vi "eyecat MAX v02_JS_140210.vi"() -> ()   [LabVIEW 2014]
doc: "This VI is an upgrade from the WIN 1_v4 that implements the ageing subrutine"
uses:
  Buttons/String output.ctl
  <vilib>/Utility/miscctls.llb/LVRowAndColumnTypeDef.ctl
  Buttons/Numeric control.ctl
  Buttons/String input.ctl
  Buttons/Numeric indicator.ctl
  Controls Win/Control 3.ctl
  <vilib>/Platform/TimedLoop/XDataNode/nitl_modes.ctl
  <vilib>/Platform/TimedLoop/XDataNode/timing_clust.ctl
  <vilib>/Platform/TimedLoop/XDataNode/wakeup.ctl
  <vilib>/Utility/file.llb/Read From Spreadsheet File (DBL).vi
  <vilib>/Utility/file.llb/Write To Spreadsheet File (string).vi
  <vilib>/Utility/file.llb/Read From Spreadsheet File (string).vi
  <vilib>/regexp/Match Regular Expression.xnode
  <vilib>/Platform/TimedLoop/XDataNode/XDataNode.xnode
  <vilib>/Platform/TimedLoop/XDataNode/XDNodeRunTimeDep.lvlib
panel:
  out "HC Cyc 2 Array":dbl[](array[numeric])
  out "SO Valve 2 array":dbl[](array[numeric])
  out "SO Valve 1 array":dbl[](array[numeric])
  out "Air Bal array":dbl[](array[numeric])
  out "HC Bal array":dbl[](array[numeric])
  out "Air Cyc array":dbl[](array[numeric])
  out "HC Cyc array":dbl[](array[numeric])
  out "File name":string
  out "Log?":bool
  out "Advanced Logging":bool
  out "output cluster":T2
  out "Connected":bool
  out "MKS 1":i16
  out "MKS 2":i16
  out "Furnace temp 2":dbl
  out "Full system?":bool
  out "Log interval (seconds)":T1
  in  "Flow rate Age":dbl
  in  "Inlet temp Age":dbl
  out "Stopped?":bool
  in  "Stop Cmd":T1
  out "Connected?":bool
  out "Error":dbl
  out "Iteration Duration":i64
  out "Finished Late? [i-1]":bool
  in  "stop TCP":bool
  in  "SO2 ppm":dbl
  out "Furnace temp 1":dbl
  out "stop 2":bool
  in  "Enum 1":i16=1
  in  "Acknowledge":bool
  out "Test number":u16
  out "Flag1":bool=TRUE
  out "EditPos Subc":T3
  out "Flag 2":bool=TRUE
  in  "Tab Control":T4(tab)
  out "Doors Unlocked":bool
  in  "Temperature Limit (°C)":T1=800.0 min=0.0 max=1200.0 step=1.0
  in  "Log Test Button":bool
  in  "File Name":T5="Test"
  in  "File Path":path=path "C:/DATA LOG"
  out "Fail":bool
  out "Pass":bool
  in  "Select Test Type":T6(radio)
  out "Standby":bool
  out "Doors Open":bool
  out "Extractor Fan On":bool
  out "Test In Progress":bool
  out "Cool Down":bool
  out "System Alarm":bool
  in  "Execute Leak Test Button":bool
  in  "Stop Test Button":bool
  in  "Start Test Button":bool
  in  "Advanced settings":bool
  in  "Inlet Temperature (°C)":T1=400.0 min=350.0 max=1000.0 step=1.0
  in  "Inlet LAMBDA Rich":T1=0.9 min=0.85 max=0.96 step=0.001
  in  "Inlet LAMBDA Lean":T1=1.2 min=1.02 max=3.0 step=0.001
  in  "Test Stop temperature (°C)":T1=300.0 min=100.0 max=1000.0 step=1.0
  in  "Test Start Temperature (°C)":T1=125.0 min=0.0 max=500.0 step=1.0
  in  "Furnace Ramp Rate (°C/min)":T1=15.0 min=1.0 max=50.0 step=0.1
  in  "NO:CO Ratio":T1=1.1 min=1.0 max=5.0 step=0.1
  in  "Inlet O2 (%)":T1=0.5 min=0.0 max=14.0 step=0.01
  in  "Inlet LAMBDA":T1=1.0 min=0.6 max=3.0 step=0.001
  out "Space Velocity (h-1)":T7
  out "Vol Flow @ STP (l/min)":T7
  in  "Test Flow Rate(g/s)":T1 min=0.0 max=100.0 step=0.01
  out "Sample Volume (litres)":T7
  in  "Number of Samples":T1=1.0 min=1.0 max=6.0 step=1.0
  in  "Sample Diameter (mm)":T1
  out "CO Theory (%)":T7 format="%#_3g"
  out "CO Theory (%)":T7 format="%#_3g"
  out "HC Theory (%)":T7
  in  "Sample Length (mm)":T1 min=0.0 step=0.5
  in  "NO ppm SW":dbl=500.0 caption="NO (ppm)" min=0.0 max=500.0 step=1.0
  in  "NO ppm Loff":T1 caption="NO ppm"
  in  "Delete sCycle":bool
  in  "Load sCycle":bool
  in  "Save sCycle":bool
  in  "Clear subcycle":bool
  in  "Clear Cycle Pattern":bool
  in  "Save Cycle":bool
  in  "Load Cycle":bool
  in  "Delete Cycle":bool
  out "Test Compiled":bool
  in  "Compile Test Button":bool
  in  "Sub-Cycle List":i32(listbox)=1
  in  "Cycle List":i32(listbox)=2
  out "Total Test Duration (hrs)":T8
  in  "Ageing Gas":enum32{"Radio Selection 1", "Radio Selection 2"}(radio)
  in  "Sub-Cycle Pattern":string[][](table) caption="Subcycle pattern"
  in  "Total Number of Cycles":T1=1.0 min=1.0 max=10000.0 step=1.0
  in  "Cycle Pattern":string[][](table)
  in  "Sub-Cycle Name":T5
  in  "Cycle Name":T5
  out "Heat Exchanger Temperatures (°C)":dynamicdata(graph)
  out "Flow Rate (g/s)":dynamicdata(graph)
  out "Sample Temperatures (°C)":dynamicdata(graph)
  out "System Temperatures (°C)":dynamicdata(graph)
  out "HC Concentration (ppm)":dynamicdata(graph)
  out "Lambda":dynamicdata(graph)
  out "M584L Upstream & Downstream":dynamicdata(graph)
  out "NO Concentration (ppm)":dynamicdata(graph)
  in  "Purge System":bool
  in  "Alarm ack":bool
  in  "Clear log":bool
  out "Table":string[][](table)
  out "Soft Alarm":bool
  out "Hard Alarm":bool
  # "Test Type"
  # "Test Commands"
  # "System Indicators"
  # "Leak Test"
  # "Catalyst Specification"
  # "Lightoff Settings"
  # "Furnace Lightoff Settings"
  # "Sweep Settings"
  # "CO/HC Lightoff Settings"
  # "0.96 < lambda < 0.85"
  # "1.02< lambda < 1.6"
  # "350 < Tinlet < 1000"
  # "NO Lightoff Settings"
  # "Flow Specification"
  # "Cycle Compiled"
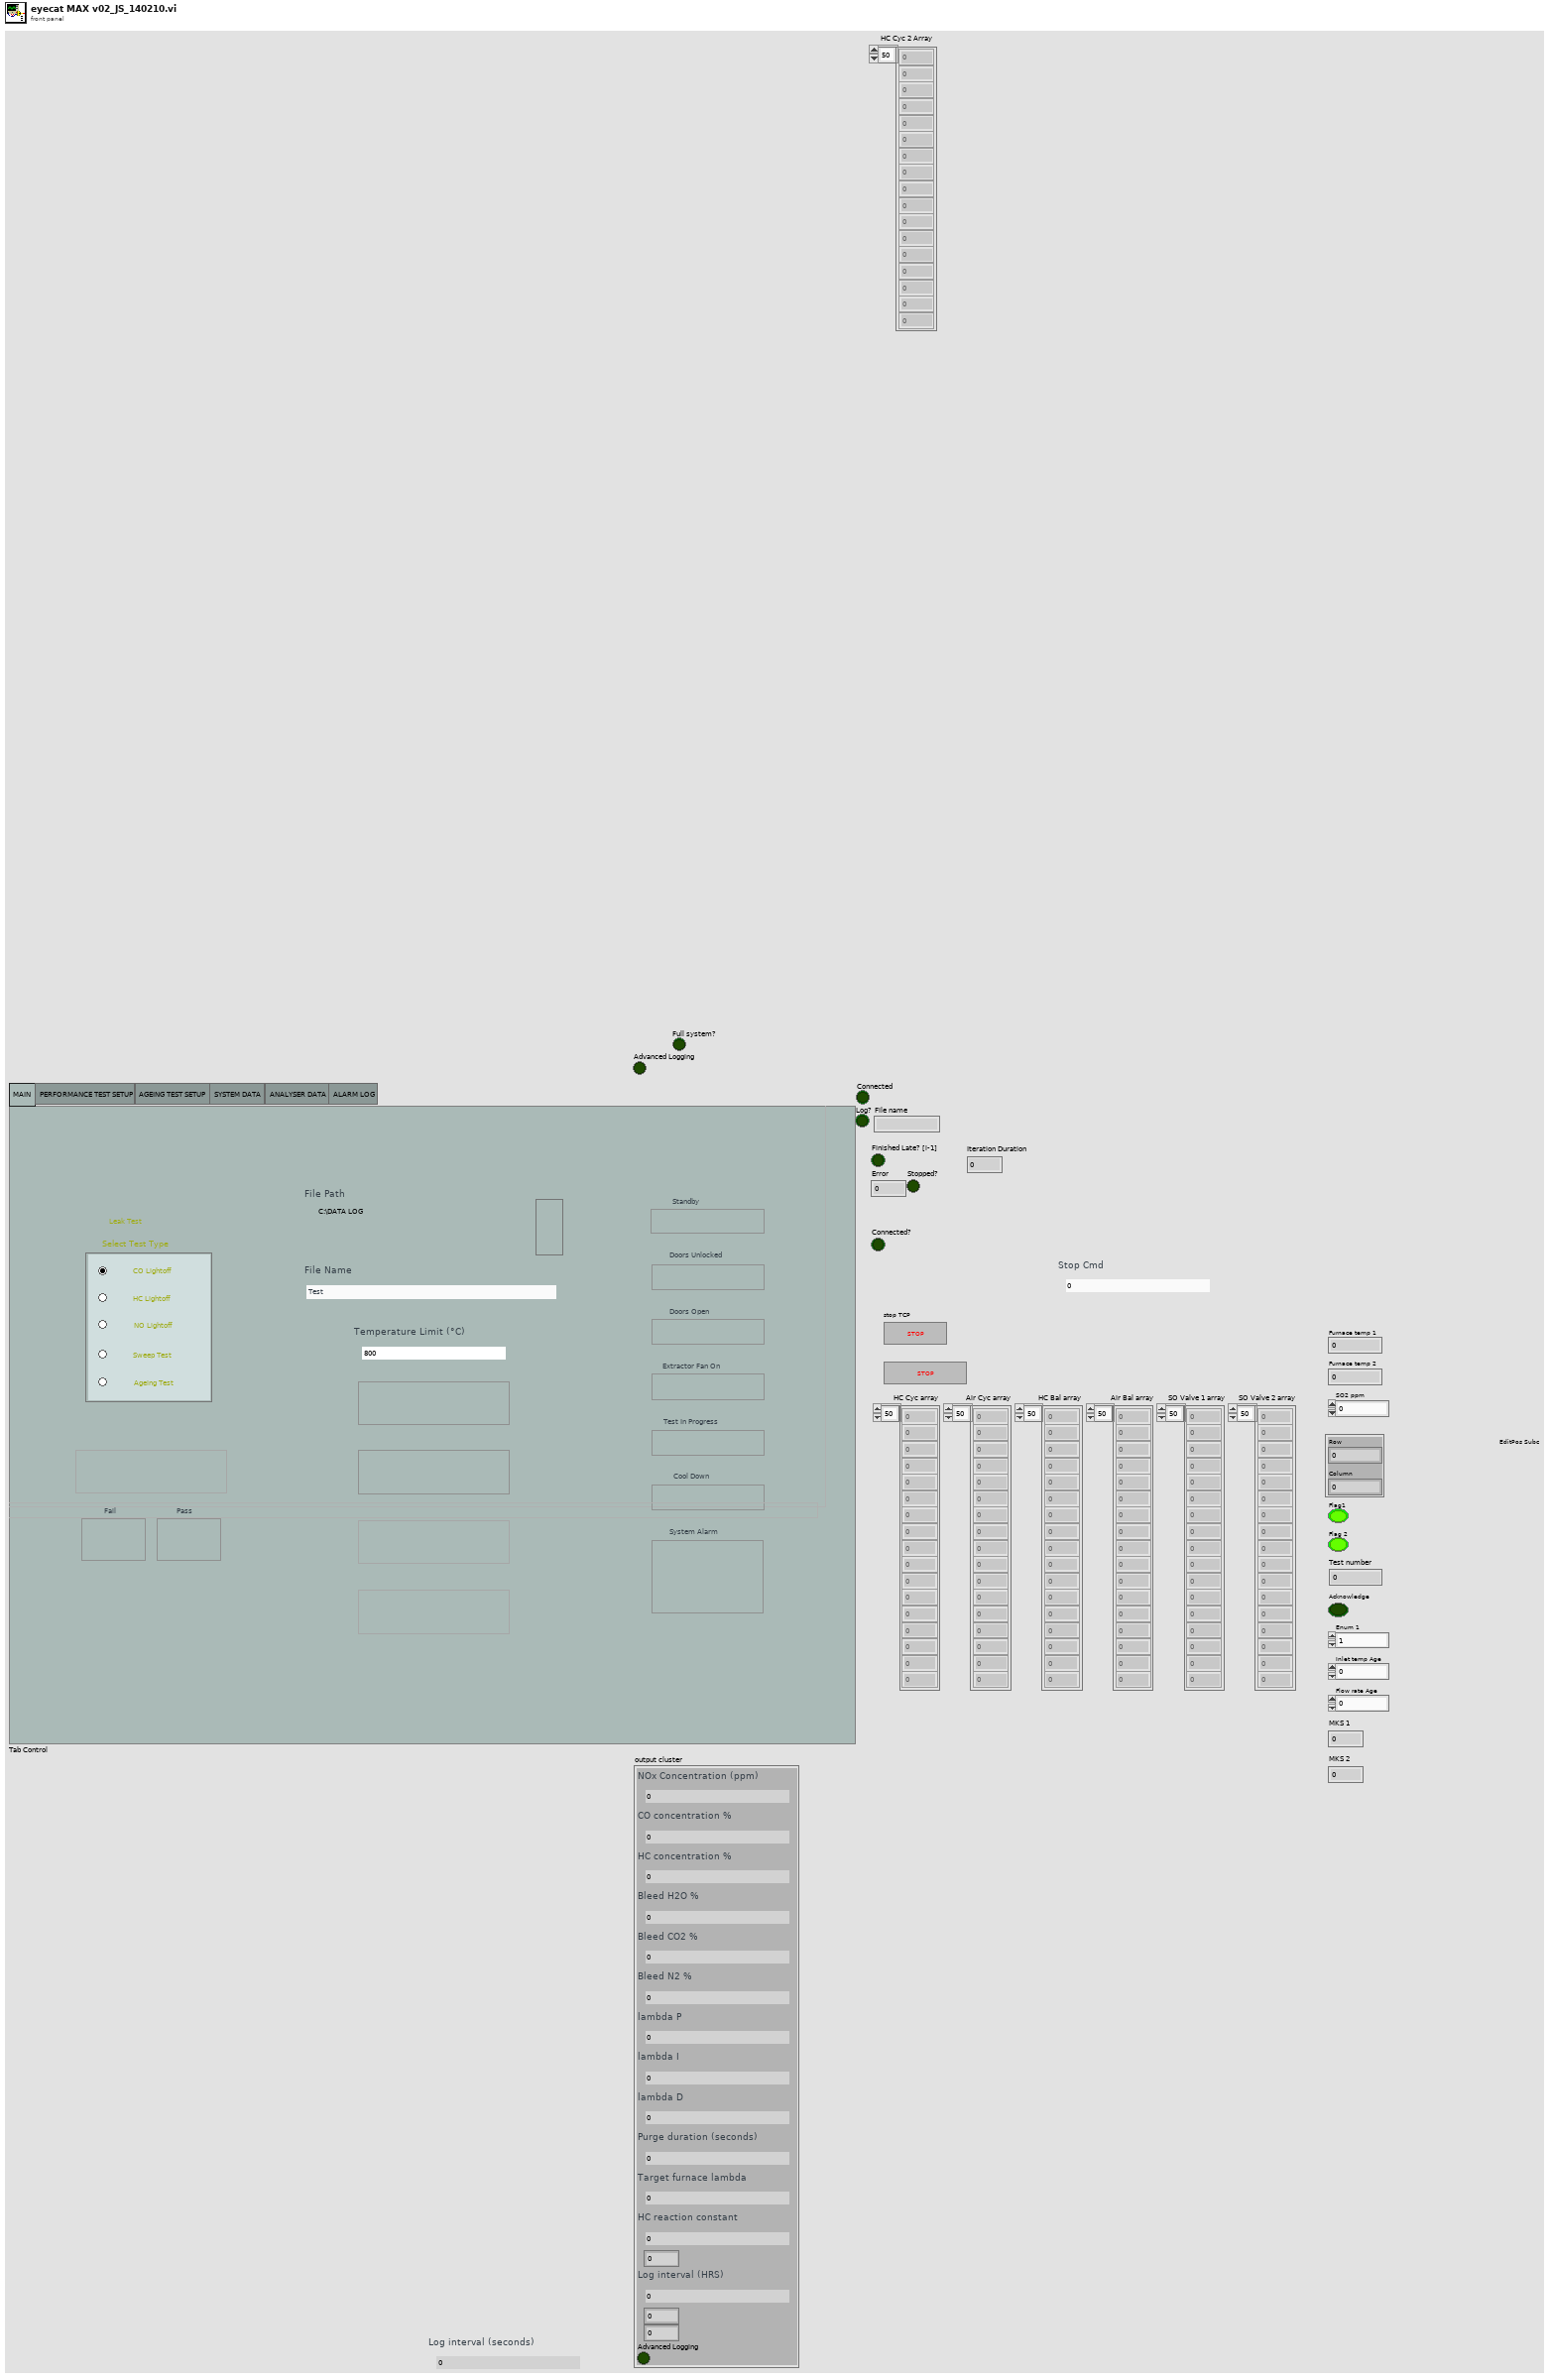
[diagram p1: front panel]
types:
  T1 = typedef "Numeric control.ctl" = dbl
  T2 = cluster{"NOx Concentration (ppm)":T1, "CO concentration %":T1, "HC concentration %":T1, "Bleed H2O %":T1, "Bleed CO2 %":T1, "Bleed N2 %":T1, "lambda P":T1, "lambda I":T1, "lambda D":T1, "Purge duration (seconds)":T1, "Target furnace lambda":T1, "HC reaction constant":T1, i16, "Log interval (HRS)":T1, i16, i16, "Advanced Logging":bool}
  T3 = typedef "LVRowAndColumnTypeDef.ctl" = cluster{"Row":i32, "Column":i32}
  T4 = enum32{"MAIN", "PERFORMANCE TEST SETUP", "AGEING TEST SETUP", "SYSTEM DATA", "ANALYSER DATA", "ALARM LOG"}
  T5 = typedef "String input.ctl" = string
  T6 = enum32{"CO Lightoff", "HC Lightoff", "NO Lightoff", "Sweep Test", "Ageing Test"}
  T7 = typedef "Numeric indicator.ctl" = dbl
  T8 = typedef "String output.ctl" = string
  T9 = typedef "XDNodeRunTimeDep.lvlib/nitl_modes.ctl" = enum32{"No Change", "Process missed periods, maintain original phase", "Discard missed periods, maintain original phase", "Process missed periods, ignore original phase", "Discard missed periods, ignore original phase"}
  T10 = typedef "Control 3.ctl" = enum16{"main", "start test", "save subc", "load subc", "delete subc", "clear table 1", "update list 1", "save cycle", "load cycle", "delete cycle", "clear table 2", "update list 2", "calc HC CO", "Total time calc", "update Cycle pattern ", "load cycle name", "convert to num", "load test array", "check scycle name", "check cycle name", "Multigas connect", "Multigas disconnect"}
  T11 = enum8{"Enabled", "Disabled", "Disabled and Grayed Out"}
  T12 = typedef "XDNodeRunTimeDep.lvlib/timing_clust.ctl" = cluster{"Expected End [f-1]":u64, "Actual End [f-1]":u64, "Finished Late? [f-1]":bool, "Expected End [i-1]":u64, "Actual End [i-1]":u64, "Finished Late? [i-1]":bool, "Expected Start [i]":u64, "Actual Start [i]":u64, "Expected Start [f]":u64, "Actual Start [f]":u64, "Source Name":string, "Structure Name":string, "Period":i64, "Deadline":i64, "Offset":i64, "Start":i64, "Priority":i32, "Timeout":i32, "Mode":T9, "Wakeup Reason":T13, "Error":errorcluster, "Source Type":string, "Secondary Source Type":string, "Global End Time":u64, "Global Start Time":u64, "Frame Duration":u64, "Iteration Duration":u64, "Assigned CPU":i32, "I/O Scan Engine Mode":u32}
  T13 = typedef "XDNodeRunTimeDep.lvlib/wakeup.ctl" = enum32{"Normal", "Aborted", "Asynchronous wakeup", "Timing source error", "Timed loop error", "Timeout"}
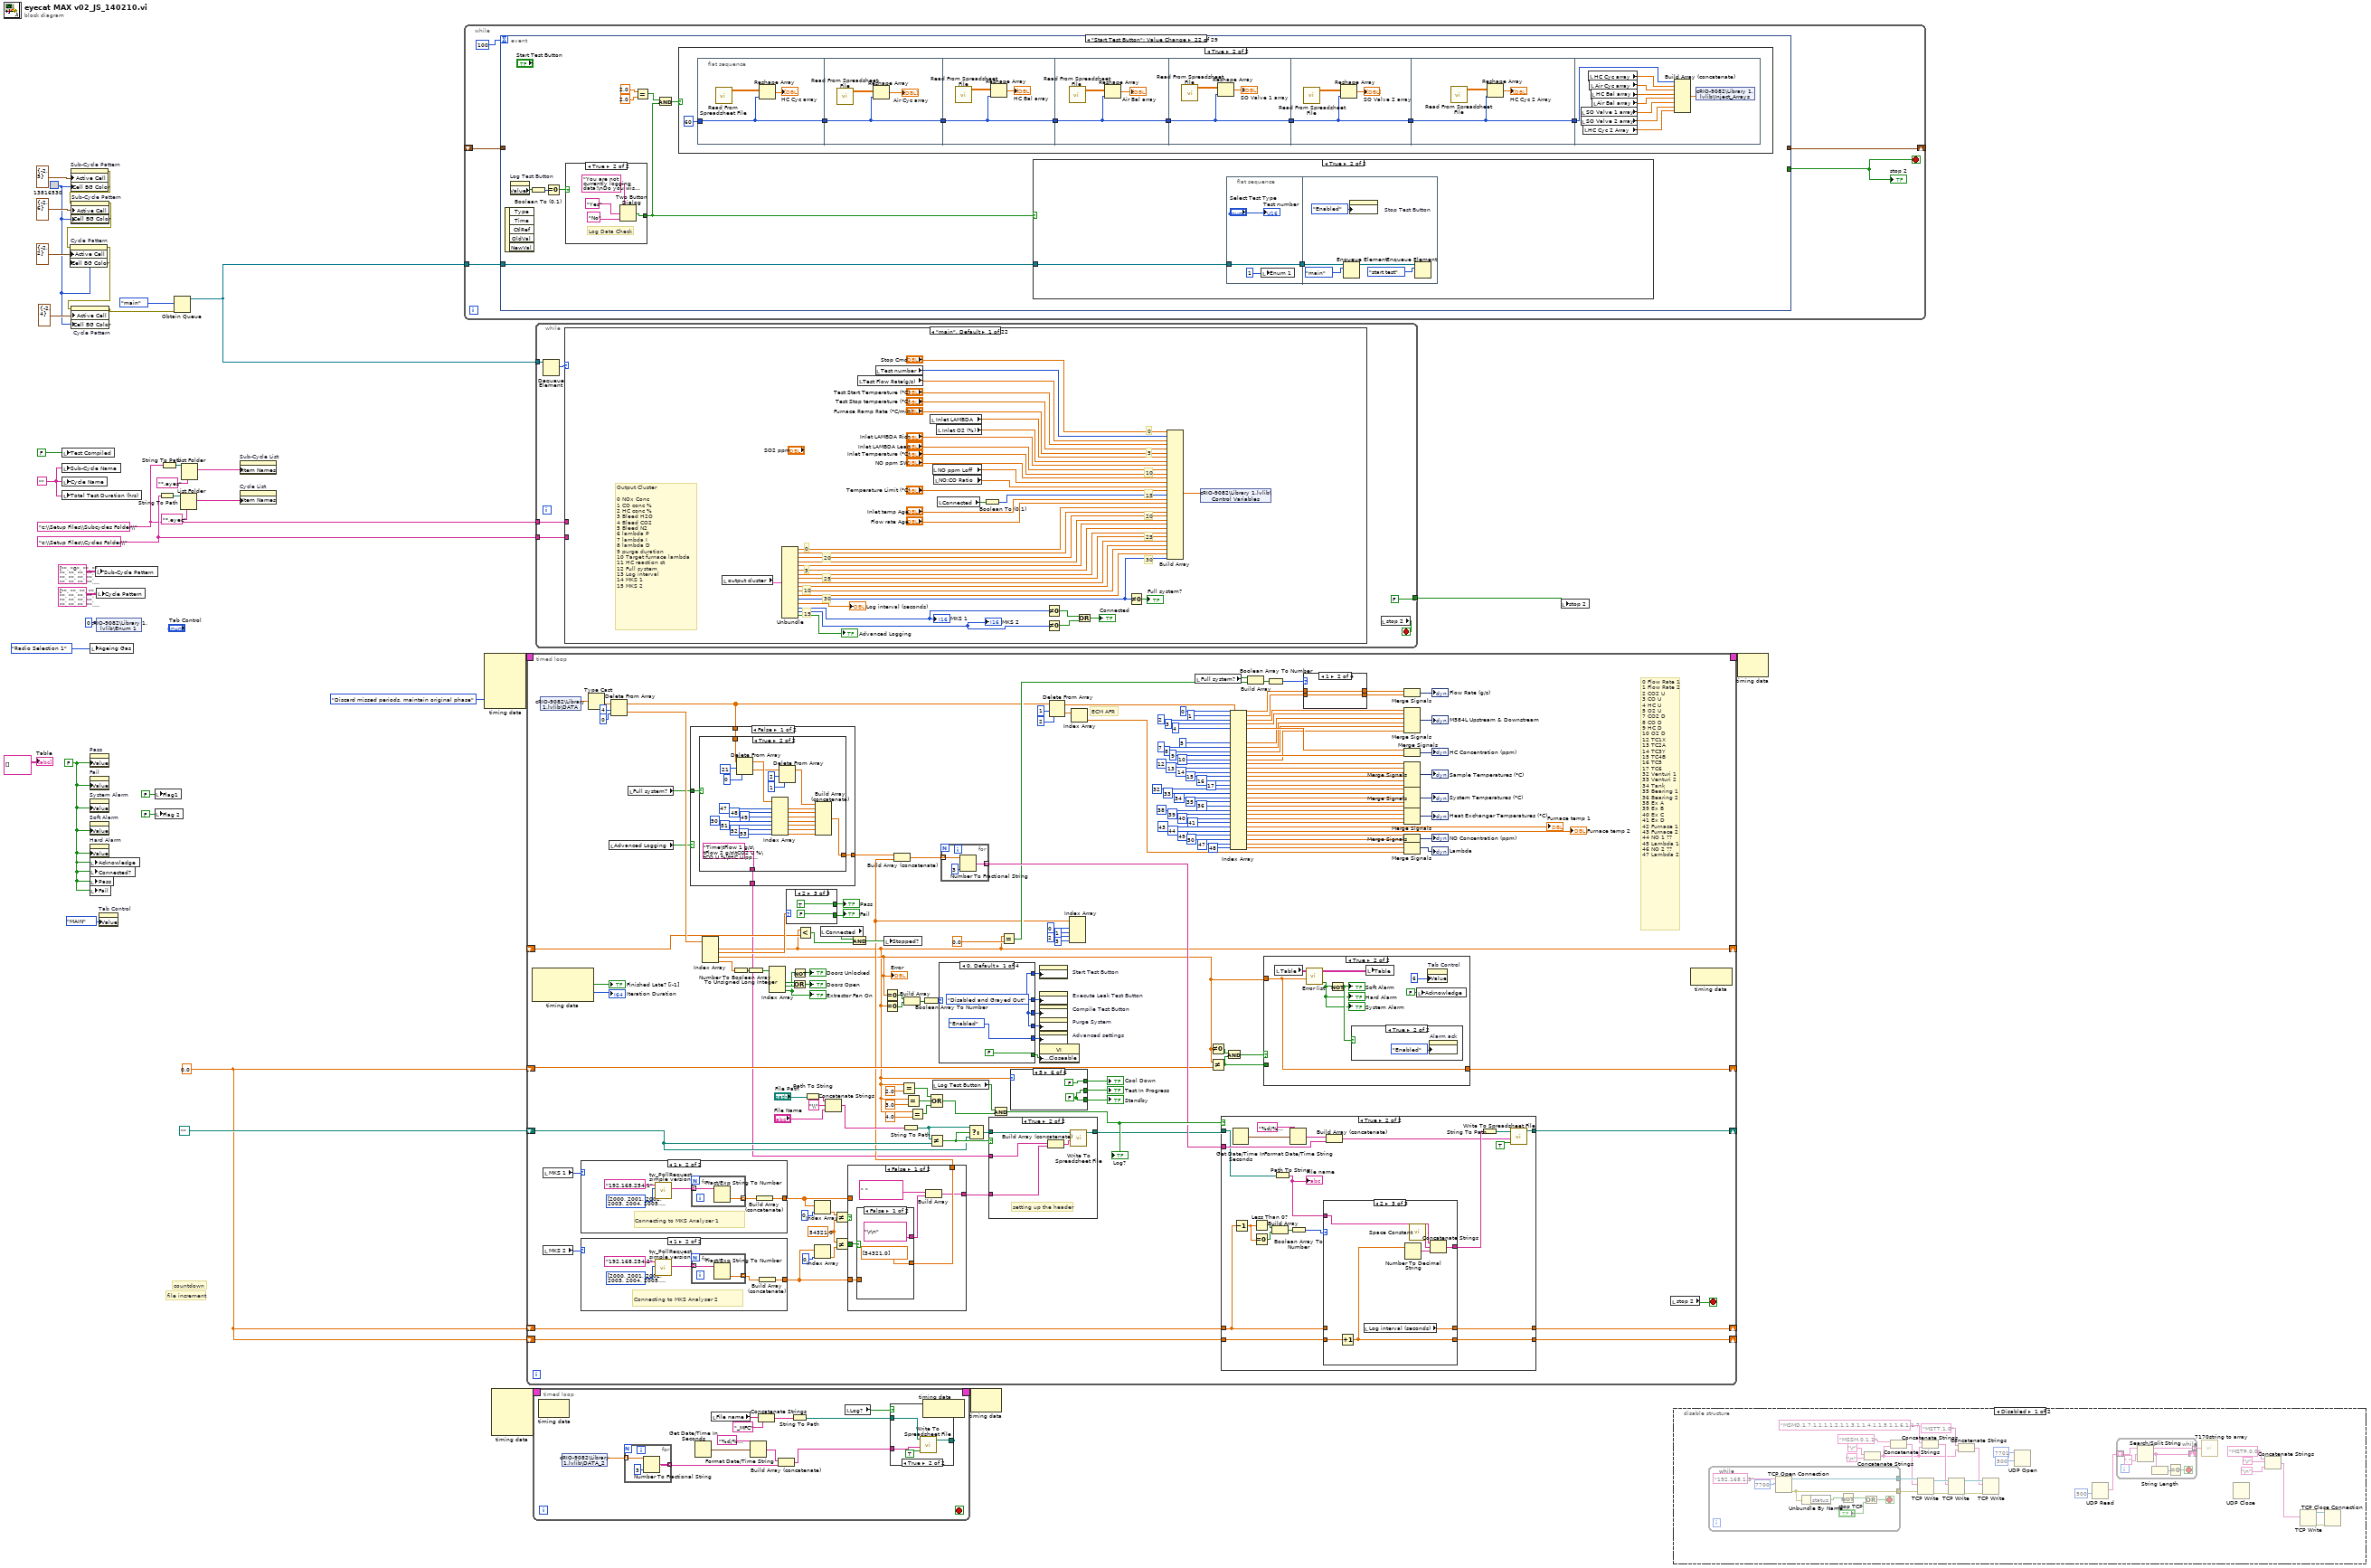
[diagram p0: block diagram]
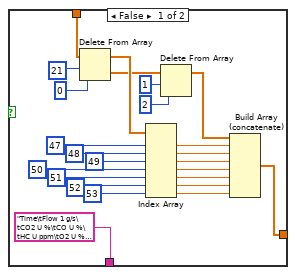
[diagram p4: hidden frame]
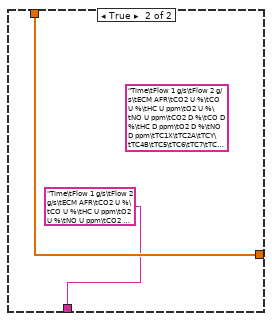
[diagram p5: hidden frame]
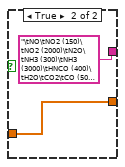
[diagram p6: hidden frame]
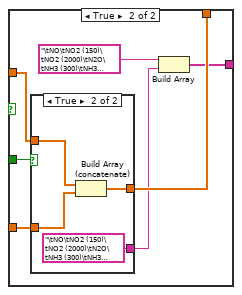
[diagram p7: hidden frame]
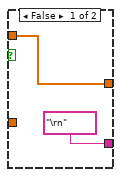
[diagram p8: hidden frame]
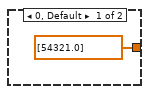
[diagram p9: hidden frame]
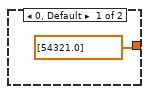
[diagram p10: hidden frame]
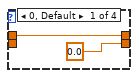
[diagram p11: hidden frame]
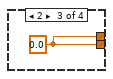
[diagram p12: hidden frame]
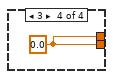
[diagram p13: hidden frame]
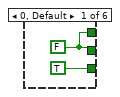
[diagram p14: hidden frame]
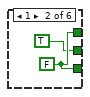
[diagram p15: hidden frame]
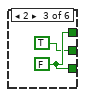
[diagram p16: hidden frame]
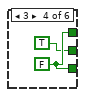
[diagram p17: hidden frame]
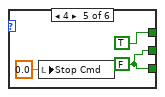
[diagram p18: hidden frame]
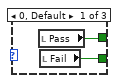
[diagram p19: hidden frame]
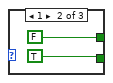
[diagram p20: hidden frame]
diagram:
  w4 = FALSE
  w3 = 0.0 ("y")
  w20 = ""
  w23 = "c:\\Setup Files\\Cycles Folder\\"
  w29 = u32 13816530
  w21 = "c:\\Setup Files\\Subcycles Folder\\"
  # "file increment"
  # "countdown"
  n1 = local write "Test Compiled"(FALSE ("Cycle Compiled")) -> ()
  n2 = local write "Sub-Cycle Name"(w20) -> ()
  n3 = local write "Cycle Name"(w20) -> ()
  n4 = local write "Total Test Duration (hrs)"(w20) -> ()
  n5 = property on="Sub-Cycle Pattern" class="Tbl (strict)"("Active Cell"=T3 {"Row"=-2, "Column"=5} ("Active Cell:Active Cell"), "Cell BG Color"=w29) -> (error out=w34:errorcluster)  [unwired: 2 in, 1 out]
  n6 = property on="Sub-Cycle Pattern" class="Tbl (strict)"(error in=w34, "Active Cell"=T3 {"Row"=-2, "Column"=6} ("Active Cell:Active Cell"), "Cell BG Color"=w29) -> (error out=w33:errorcluster)  [unwired: 1 in, 1 out]
  n7 = property on="Cycle Pattern" class="Tbl (strict)"(error in=w33, "Active Cell"=T3 {"Row"=-2, "Column"=2} ("Active Cell:Active Cell"), "Cell BG Color"=w29) -> (error out=w31:errorcluster)  [unwired: 1 in, 1 out]
  n8 = property on="Cycle Pattern" class="Tbl (strict)"(error in=w31, "Active Cell"=T3 {"Row"=-2, "Column"=4} ("Active Cell:Active Cell"), "Cell BG Color"=w29) -> (error out=w28:errorcluster)  [unwired: 1 in, 1 out]
  n9 = property on="Pass" class="Bool (strict)"("Value"=w4) -> ()  [unwired: 2 in, 2 out]
  n10 = property on="Fail" class="Bool (strict)"("Value"=w4) -> ()  [unwired: 2 in, 2 out]
  n11 = property on="System Alarm" class="Bool (strict)"("Value"=w4) -> ()  [unwired: 2 in, 2 out]
  n12 = property on="Soft Alarm" class="Bool (strict)"("Value"=w4) -> ()  [unwired: 2 in, 2 out]
  n13 = property on="Hard Alarm" class="Bool (strict)"("Value"=w4) -> ()  [unwired: 2 in, 2 out]
  n14 = local write "Acknowledge"(w4) -> ()
  n15 = local write "Connected?"(w4) -> ()
  n16 = local write "Pass"(w4) -> ()
  n17 = local write "Fail"(w4) -> ()
  n18 = local write "Ageing Gas"(enum32{"Radio Selection 1", "Radio Selection 2"}."Radio Selection 1" ("Ageing Gas")) -> ()
  n19 = local write "Sub-Cycle Pattern"(string[][] [["", "0", "", "", "", "", "", "", "", "", "", "", ""], ["", "", "", "", "", "", "", "", "", "", "", "", ""], ["", "", "", "", "", "", "", "", "", "", "", "", ""], ["", "", "", "", "", "", "", "", "", "", "", "", ""], ["", "", "", "", "", "", "", "", "", "", "", "", ""], ["", "", "", "", "", "", "", "", "", "", "", "", ""], ["", "", "", "", "", "", "", "", "", "", "", "", ""], ["", "", "", "", "", "", "", "", "", "", "", "", ""], ["", "", "", "", "", "", "", "", "", "", "", "", ""], ["", "", "", "", "", "", "", "", "", "", "", "", ""], ["", "", "", "", "", "", "", "", "", "", "", "", ""], ["", "", "", "", "", "", "", "", "", "", "", "", ""], ["", "", "", "", "", "", "", "", "", "", "", "", ""], ["", "", "", "", "", "", "", "", "", "", "", "", ""], ["", "", "", "", "", "", "", "", "", "", "", "", ""], ["", "", "", "", "", "", "", "", "", "", "", "", ""], ["", "", "", "", "", "", "", "", "", "", "", "", ""], ["", "", "", "", "", "", "", "", "", "", "", "", ""], ["", "", "", "", "", "", "", "", "", "", "", "", ""], ["", "", "", "", "", "", "", "", "", "", "", "", ""], ["", "", "", "", "", "", "", "", "", "", "", "", ""], ["", "", "", "", "", "", "", "", "", "", "", "", ""], ["", "", "", "", "", "", "", "", "", "", "", "", ""], ["", "", "", "", "", "", "", "", "", "", "", "", ""], ["", "", "", "", "", "", "", "", "", "", "", "", ""], ["", "", "", "", "", "", "", "", "", "", "", "", ""], ["", "", "", "", "", "", "", "", "", "", "", "", ""], ["", "", "", "", "", "", "", "", "", "", "", "", ""], ["", "", "", "", "", "", "", "", "", "", "", "", ""], ["", "", "", "", "", "", "", "", "", "", "", "", ""], ["", "", "", "", "", "", "", "", "", "", "", "", ""]]) -> ()
  n20 = local write "Cycle Pattern"(string[][] [["", "", "", "", ""], ["", "", "", "", ""], ["", "", "", "", ""], ["", "", "", "", ""], ["", "", "", "", ""], ["", "", "", "", ""], ["", "", "", "", ""], ["", "", "", "", ""], ["", "", "", "", ""], ["", "", "", "", ""], ["", "", "", "", ""], ["", "", "", "", ""], ["", "", "", "", ""], ["", "", "", "", ""], ["", "", "", "", ""], ["", "", "", "", ""], ["", "", "", "", ""], ["", "", "", "", ""], ["", "", "", "", ""], ["", "", "", "", ""], ["", "", "", "", ""], ["", "", "", "", ""], ["", "", "", "", ""], ["", "", "", "", ""], ["", "", "", "", ""], ["", "", "", "", ""], ["", "", "", "", ""], ["", "", "", "", ""], ["", "", "", "", ""], ["", "", "", "", ""], ["", "", "", "", ""]]) -> ()
  n21 = shared-variable "cRIO-9082\\Library 1.lvlib\\Enum 1"(u16 0 ("Enum 1")) -> ()  [unwired: 1 in, 1 out]
  n22 = property on="Tab Control" class="TabCtl (strict)"("Value"=T4."MAIN" ("Tab Control")) -> ()  [unwired: 2 in, 2 out]
  n23 = local write "Flag1"(FALSE) -> ()
  n24 = local write "Flag 2"(FALSE) -> ()
  n25 = String To Path(string=w23) -> (path=w24:path)
  n26 = String To Path(string=w21) -> (path=w26:path)
  n27 = Obtain Queue(element data type=Control_3."main" ("Enum"), error in (no error)=w28) -> (queue out=w37:refnum<queue>)  [unwired: 3 in, 2 out]
  n28 = List Folder(path=w24, pattern="*.eyec") -> (filenames=w25:string[])  [unwired: 2 in, 3 out]
  n29 = List Folder(path=w26, pattern="*.eyes") -> (filenames=w27:string[])  [unwired: 2 in, 3 out]
  n30 = property on="Sub-Cycle List" class="LstBox (strict)"("Item Names"=w27) -> ()  [unwired: 2 in, 2 out]
  n31 = property on="Cycle List" class="LstBox (strict)"("Item Names"=w25) -> ()  [unwired: 2 in, 2 out]
  n32 = while {
    tunnel: w37 -> [w43]
    shift-right: [w41] -> _
    shift-left: _ -> [w40]
    stop <- w39 stop-if-true
    n33 = event shown="[21] \"Start Test Button\": Value Change" {
      selector: _ -> [_ _ _ _ _ _ _ _ _ _ _ _ _ _ _ _ _ _ _ _ _ _ _ _ _ _ _ _ _]
      dyn-events: _ -> [_ _ _ _ _ _ _ _ _ _ _ _ _ _ _ _ _ _ _ _ _ _ _ _ _ _ _ _ _]
      timeout: 100 -> [_ _ _ _ _ _ _ _ _ _ _ _ _ _ _ _ _ _ _ _ _ _ _ _ _ _ _ _ _]
      tunnel: w43 -> [w46 w48 _ w57 w65 w72 w79 w90 w94 w105 w110 w113 w118 w140 w148 w149 _ _ _ _ w193 w209 _ w272 w290 _ w304 _ _]
      tunnel: [w44 w47 _ w58 w64 w71 w78 w89 w92 w100 w107 w112 w116 w137 _ _ _ _ _ _ _ _ _ _ _ _ _ _ _] -> w41
      tunnel: w40 -> [w44 w47 _ w58 w64 w71 w77 w89 w92 w100 w107 w112 w116 w137 _ _ _ _ _ _ _ _ _ _ _ _ _ _ _]
      tunnel: [_ _ w50 _ _ _ _ _ _ _ _ _ _ _ _ _ _ _ _ _ _ _ _ _ _ _ _ _ _] -> w39
      event Timeout {
        n34 = event-data() -> ()  [unwired: 1 in, 2 out]
        n35 = Enqueue Element(queue=w46, element=Control_3."main" ("Enum")) -> ()  [unwired: 2 in, 3 out]
      }
      event "Clear subcycle": Value Change {
        n36 = event-data() -> ()  [unwired: 1 in, 5 out]
        n37 = Enqueue Element(queue=w48, element=Control_3."clear table 1" ("Enum")) -> ()  [unwired: 2 in, 3 out]
      }
      event Panel Close? {
        n38 = event-data() -> ()  [unwired: 1 in, 3 out]
        n39 = Two Button Dialog(message="This command will close Eyecat!\nDo you wish to continue?", 1:"No" ("F button name (\"Cancel\")"), 2:"Yes" ("T button name (\"OK\")")) -> (T button?=w50:bool)
        n40 = Not(x=w50) -> (.not. x?=w51:bool)
        n41 = event-data("Discard?"=w51) -> ()  [unwired: 1 in, 1 out]
      }
      event "Save sCycle": Value Change {
        n42 = event-data() -> ()  [unwired: 1 in, 5 out]
        n43 = local read "Sub-Cycle Pattern"() -> (w55:string[][])
        n44 = call "Time column check.vi"("Array"=w55) -> ("Mistake?"=w56:bool)  [unwired: 10 in]
        n45 = case shown="False" w56 {
          tunnel: w57 -> [w59 _]
          frame False {
            n46 = Enqueue Element(queue=w59, element=Control_3."save subc") -> (queue out=w61:refnum<queue>)  [unwired: 2 in, 2 out]
            n47 = Enqueue Element(queue=w61, element=Control_3."update list 1") -> ()  [unwired: 2 in, 3 out]
          }
          frame True {
            n48 = One Button Dialog(message="The time sequence is incorrect!\nReview and save again!") -> ()  [unwired: 1 in, 1 out]
          }
        }
      }
      event "Load sCycle": Value Change {
        n49 = event-data() -> ()  [unwired: 1 in, 5 out]
        n50 = Enqueue Element(queue=w65, element=Control_3."load subc") -> ()  [unwired: 2 in, 3 out]
      }
      event "Delete sCycle": Value Change {
        n51 = event-data() -> ()  [unwired: 1 in, 5 out]
        n52 = Enqueue Element(queue=w72, element=Control_3."delete subc") -> (queue out=w74:refnum<queue>)  [unwired: 2 in, 2 out]
        n53 = Enqueue Element(queue=w74, element=Control_3."update list 1") -> (queue out=w70:refnum<queue>)  [unwired: 2 in, 2 out]
        n54 = Enqueue Element(queue=w70, element=Control_3."update Cycle pattern ") -> (queue out=w67:refnum<queue>)  [unwired: 2 in, 2 out]
        n55 = Enqueue Element(queue=w67, element=Control_3."Total time calc") -> ()  [unwired: 2 in, 3 out]
      }
      event "Sub-Cycle Pattern": Mouse Down; "Sub-Cycle Pattern": Value Change {
        n56 = event-data() -> ()  [unwired: 1 in, 3 out]
        n57 = property on="Sub-Cycle Pattern" class="Tbl (strict)"() -> ("EditPos"=w78:T3)  [unwired: 2 in, 2 out]
        n58 = Unbundle By Name(w78) -> ("Row"=w80:i32)  [unwired: 1 out]
        n59 = Less?(x=w80, y=30) -> (x < y?=w82:bool)
        n60 = case shown="True" w82 {
          tunnel: w79 -> [_ w87]
          frame False {
            n61 = One Button Dialog(message="This table is limited to 30 entries!") -> ()  [unwired: 1 in, 1 out]
          }
          frame True {
            n62 = Enqueue Element(queue=w87, element=Control_3."convert to num") -> (queue out=w86:refnum<queue>)  [unwired: 2 in, 2 out]
            n63 = Enqueue Element(queue=w86, element=Control_3."calc HC CO") -> ()  [unwired: 2 in, 3 out]
          }
        }
        "EditPos Subc" <- w77
        "Flag1" <- TRUE
      }
      event "Clear Cycle Pattern": Value Change {
        n64 = event-data() -> ()  [unwired: 1 in, 5 out]
        n65 = Enqueue Element(queue=w90, element=Control_3."clear table 2" ("Enum")) -> ()  [unwired: 2 in, 3 out]
        n66 = local write "Test Compiled"(FALSE ("Test Compiled")) -> ()
      }
      event "Save Cycle": Value Change {
        n67 = event-data() -> ()  [unwired: 1 in, 5 out]
        n68 = Enqueue Element(queue=w94, element=Control_3."update Cycle pattern ") -> (queue out=w93:refnum<queue>)  [unwired: 2 in, 2 out]
        n69 = Enqueue Element(queue=w93, element=Control_3."save cycle") -> (queue out=w97:refnum<queue>)  [unwired: 2 in, 2 out]
        n70 = Enqueue Element(queue=w97, element=Control_3."update list 2") -> ()  [unwired: 2 in, 3 out]
      }
      event "Load Cycle": Value Change {
        n71 = event-data() -> ()  [unwired: 1 in, 5 out]
        n72 = Enqueue Element(queue=w105, element=Control_3."load cycle") -> (queue out=w103:refnum<queue>)  [unwired: 2 in, 2 out]
        n73 = Enqueue Element(queue=w103, element=Control_3."update Cycle pattern ") -> (queue out=w102:refnum<queue>)  [unwired: 2 in, 2 out]
        n74 = local write "Test Compiled"(FALSE ("Test Compiled")) -> ()
        n75 = Enqueue Element(queue=w102, element=Control_3."Total time calc") -> ()  [unwired: 2 in, 3 out]
      }
      event "Delete Cycle": Value Change {
        n76 = event-data() -> ()  [unwired: 1 in, 5 out]
        n77 = Enqueue Element(queue=w110, element=Control_3."delete cycle") -> (queue out=w109:refnum<queue>)  [unwired: 2 in, 2 out]
        n78 = Enqueue Element(queue=w109, element=Control_3."update list 2") -> ()  [unwired: 2 in, 3 out]
      }
      event Value Change {
        n79 = event-data() -> ()  [unwired: 1 in, 5 out]
        n80 = Enqueue Element(queue=w113, element=Control_3."Total time calc") -> ()  [unwired: 2 in, 3 out]
      }
      event "Cycle Pattern": Mouse Up; "Cycle Pattern": Value Change {
        n81 = event-data() -> ()  [unwired: 1 in, 3 out]
        n82 = property on="Cycle Pattern" class="Tbl (strict)"() -> ("EditPos"=w120:T3)  [unwired: 2 in, 2 out]
        n83 = Unbundle By Name(w120) -> ("Row"=w117:i32, "Column"=w122:i32)
        n84 = Less?(x=w117, y=30) -> (x < y?=w121:bool)
        n85 = case shown="True" w121 {
          tunnel: w122 -> [_ w124]
          tunnel: w118 -> [_ w127]
          frame False {
            n86 = One Button Dialog(message="This table is limited to 30 entries!") -> ()  [unwired: 1 in, 1 out]
          }
          frame True {
            n87 = Equal?(x=w124, y=1) -> (x = y?=w128:bool)
            n88 = case shown="True" w128 {
              tunnel: w127 -> [w131 w134]
              tunnel: [w130 w133] -> w126
              frame False {
                n89 = Enqueue Element(queue=w131, element=Control_3."update Cycle pattern ") -> (queue out=w130:refnum<queue>)  [unwired: 2 in, 2 out]
              }
              frame True {
                n90 = Enqueue Element(queue=w134, element=Control_3."load cycle name") -> (queue out=w133:refnum<queue>)  [unwired: 2 in, 2 out]
              }
            }
            n91 = Enqueue Element(queue=w126, element=Control_3."Total time calc") -> ()  [unwired: 2 in, 3 out]
          }
        }
        "Flag 2" <- TRUE
      }
      event "Compile Test Button": Value Change {
        n92 = event-data() -> ()  [unwired: 1 in, 5 out]
        n93 = local read "Flag 2"() -> (w136:bool)
        n94 = case shown="True" w136 {
          tunnel: w140 -> [w141 w145]
          tunnel: [w141 w142] -> w138
          frame False {
          }
          frame True {
            n95 = Enqueue Element(queue=w145, element=Control_3."save cycle") -> (queue out=w143:refnum<queue>)  [unwired: 2 in, 2 out]
            n96 = Enqueue Element(queue=w143, element=Control_3."update list 2") -> (queue out=w142:refnum<queue>)  [unwired: 2 in, 2 out]
          }
        }
        n97 = Enqueue Element(queue=w138, element=Control_3."load test array") -> ()  [unwired: 2 in, 3 out]
      }
      event Value Change {
        n98 = event-data() -> ()  [unwired: 1 in, 5 out]
        n99 = Enqueue Element(queue=w148, element=Control_3."check scycle name") -> ()  [unwired: 2 in, 3 out]
      }
      event Value Change {
        n100 = event-data() -> ()  [unwired: 1 in, 5 out]
        n101 = Enqueue Element(queue=w149, element=Control_3."check cycle name") -> ()  [unwired: 2 in, 3 out]
      }
      event Value Change {
        n102 = event-data() -> ()  [unwired: 1 in, 5 out]
        n103 = Square(x="Sample Diameter (mm)") -> (x^2=w158:T1)
        n104 = Compound Arithmetic op=MULTIPLY(w158, "Sample Length (mm)", "Number of Samples", 3.141592653589793) -> (w157:T1)
        n105 = Divide(x=w157, y=4000000.0) -> (x/y=→"Sample Volume (litres)":T1)
      }
      event Value Change {
        # "O2Eq"
        n106 = event-data() -> ()  [unwired: 1 in, 5 out]
        n107 = local write "Inlet LAMBDA"("Inlet LAMBDA") -> ()
        n108 = local write "Inlet O2 (%)"("Inlet O2 (%)") -> ()
        n109 = Decrement(x="Inlet LAMBDA") -> (x-1=w173:T1)
        n110 = Multiply(x=4.76, y="Inlet LAMBDA") -> (x*y=w169:T1)
        n111 = Multiply(x=w173, y=100.0) -> (x*y=w171:T1)
        n112 = Add(x=0.33, y=w169) -> (x+y=w167:T1)
        n113 = Divide(x=w171, y=w167) -> (x/y=w166:T1)
        n114 = Subtract(x="Inlet O2 (%)", y=w166) -> (x-y=w164:T1)
        n115 = Multiply(x=w164, y=2.0) -> (x*y=→"CO Theory (%)":T1)
        n116 = Divide(x=w164, y=4.5) -> (x/y=→"HC Theory (%)":T1)
      }
      event Value Change {
        n117 = event-data() -> ()  [unwired: 1 in, 5 out]
        n118 = local write "NO ppm Loff"("NO ppm Loff") -> ()
        n119 = local write "NO:CO Ratio"("NO:CO Ratio") -> ()
        n120 = Divide(x="NO ppm Loff", y=T1 10000.0) -> (x/y=w176:T1)
        n121 = Multiply(x="NO:CO Ratio", y=w176) -> (x*y=→"CO Theory (%)":T1)
      }
      event Value Change {
        n122 = event-data() -> ()  [unwired: 1 in, 5 out]
        n123 = local read "Sample Volume (litres)"() -> (w181:T7)
        n124 = Equal?(x=w181, y=0.0) -> (x = y?=w180:bool)
        n125 = case shown="False" w180 {
          tunnel: w181 -> [w186 _]
          tunnel: "Test Flow Rate(g/s)" -> [w183 _]
          frame False {
            w188 = 60.0 ("y")
            n126 = Multiply(x=w183, y=w188) -> (x*y=w190:T1)
            n127 = Divide(x=w190, y=1.2) -> (x/y=w185:T1)
            "Vol Flow @ STP (l/min)" <- w185
            n128 = Multiply(x=w185, y=w188) -> (x*y=w187:T1)
            n129 = Divide(x=w187, y=w186) -> (x/y=→"Space Velocity (h-1)":T1)
          }
          frame True {
            n130 = One Button Dialog(message="Review sample specification first!") -> ()  [unwired: 1 in, 1 out]
          }
        }
      }
      event "Execute Leak Test Button": Value Change {
        n131 = event-data() -> ()  [unwired: 1 in, 5 out]
        n132 = flat-sequence {
          tunnel: w193 -> [w196]
          tunnel: [w196] -> w192
          tunnel: w192 -> [w199]
          frame #0 {
            n133 = local write "Test number"(u16 5) -> ()
            n134 = local write "Enum 1"(u16 3 ("Test number")) -> ()
          }
          frame #1 {
            n135 = Enqueue Element(queue=w199, element=Control_3."main" ("Enum")) -> (queue out=w197:refnum<queue>)  [unwired: 2 in, 2 out]
            n136 = Enqueue Element(queue=w197, element=Control_3."start test" ("Enum")) -> ()  [unwired: 2 in, 3 out]
          }
        }
      }
      event "Start Test Button": Value Change {
        n137 = event-data() -> ()  [unwired: 1 in, 5 out]
        n138 = property on="Log Test Button" class="Bool (strict)"() -> ("Value"=w208:bool)  [unwired: 2 in, 2 out]
        n139 = Boolean To (0,1)(Boolean=w208) -> (0, 1=w207:i16)
        n140 = Equal To 0?(x=w207) -> (x = 0?=w206:bool)
        n141 = case shown="True" w206 {
          tunnel: [TRUE ("T button?") w249] -> w201
          frame False {
          }
          frame True {
            # "Log Data Check"
            n142 = Two Button Dialog(message="You are not currently logging data!\nDo you wish to continue?", 1:"No" ("T button name (\"OK\")"), 2:"Yes" ("T button name (\"OK\")")) -> (T button?=w249:bool)
          }
        }
        n143 = Equal?(x=2.0, y=2.0) -> (x = y?=w202:bool)
        n144 = And(x=w202, y=w201) -> (x .and. y?=w203:bool)
        n145 = case shown="True" w203 {
          frame False {
          }
          frame True {
            n146 = flat-sequence {
              tunnel: 60 ("dimension size") -> [w218]
              tunnel: [w218] -> w216
              tunnel: w216 -> [w221]
              tunnel: [w221] -> w215
              tunnel: w215 -> [w224]
              tunnel: [w224] -> w214
              tunnel: w214 -> [w227]
              tunnel: [w227] -> w213
              tunnel: [w230] -> w217
              tunnel: w213 -> [w230]
              tunnel: [w233] -> w211
              tunnel: w217 -> [w233]
              tunnel: w211 -> [w236]
              tunnel: [w236] -> w210
              tunnel: w210 -> [w240]
              frame #0 {
                n147 = call-poly <vilib>:"Read From Spreadsheet File.vi"() -> ("all rows"=w220:dbl[][])  [unwired: 7 in, 4 out]
                n148 = Reshape Array(w220, w218) -> (→"HC Cyc array":dbl[])
              }
              frame #1 {
                n149 = call-poly <vilib>:"Read From Spreadsheet File.vi"() -> ("all rows"=w222:dbl[][])  [unwired: 7 in, 4 out]
                n150 = Reshape Array(w222, w221) -> (→"Air Cyc array":dbl[])
              }
              frame #2 {
                n151 = call-poly <vilib>:"Read From Spreadsheet File.vi"() -> ("all rows"=w226:dbl[][])  [unwired: 7 in, 4 out]
                n152 = Reshape Array(w226, w224) -> (→"HC Bal array":dbl[])
              }
              frame #3 {
                n153 = call-poly <vilib>:"Read From Spreadsheet File.vi"() -> ("all rows"=w228:dbl[][])  [unwired: 7 in, 4 out]
                n154 = Reshape Array(w228, w227) -> (→"Air Bal array":dbl[])
              }
              frame #4 {
                n155 = call-poly <vilib>:"Read From Spreadsheet File.vi"() -> ("all rows"=w232:dbl[][])  [unwired: 7 in, 4 out]
                n156 = Reshape Array(w232, w230) -> (→"SO Valve 1 array":dbl[])
              }
              frame #5 {
                n157 = call-poly <vilib>:"Read From Spreadsheet File.vi"() -> ("all rows"=w234:dbl[][])  [unwired: 7 in, 4 out]
                n158 = Reshape Array(w234, w233) -> (→"SO Valve 2 array":dbl[])
              }
              frame #6 {
                n159 = call-poly <vilib>:"Read From Spreadsheet File.vi"() -> ("all rows"=w237:dbl[][])  [unwired: 7 in, 4 out]
                n160 = Reshape Array(w237, w236) -> (→"HC Cyc 2 Array":dbl[])
              }
              frame #7 {
                n161 = local read "SO Valve 1 array"() -> (w245:dbl[])
                n162 = local read "SO Valve 2 array"() -> (w246:dbl[])
                n163 = local read "HC Cyc 2 Array"() -> (w239:dbl[])
                n164 = local read "HC Cyc array"() -> (w241:dbl[])
                n165 = local read "Air Cyc array"() -> (w242:dbl[])
                n166 = local read "HC Bal array"() -> (w243:dbl[])
                n167 = local read "Air Bal array"() -> (w244:dbl[])
                n168 = Build Array (concatenate)(w240, w241, w242, w243, w244, w245, w246, w239) -> (w247:dbl[])
                n169 = shared-variable "cRIO-9082\\Library 1.lvlib\\Inject_Arrays"(w247) -> ()  [unwired: 1 in, 1 out]
              }
            }
          }
        }
        n170 = case shown="True" w201 {
          tunnel: w209 -> [_ w254]
          frame False {
          }
          frame True {
            n171 = flat-sequence {
              tunnel: w254 -> [w257]
              tunnel: [w257] -> w253
              tunnel: w253 -> [w261]
              frame #0 {
                n172 = local write "Enum 1"(u16 1 ("Test number")) -> ()
                "Test number" <- "Select Test Type"
              }
              frame #1 {
                n173 = Enqueue Element(queue=w261, element=Control_3."main" ("Enum")) -> (queue out=w259:refnum<queue>)  [unwired: 2 in, 2 out]
                n174 = property on="Stop Test Button" class="Bool"("DisabledEnum"=T11."Enabled" ("Disabled")) -> ()  [unwired: 2 in, 2 out]
                n175 = Enqueue Element(queue=w259, element=Control_3."start test" ("Enum")) -> ()  [unwired: 2 in, 3 out]
              }
            }
          }
        }
      }
      event "Log Test Button": Value Change {
        n176 = event-data() -> ()  [unwired: 1 in, 6 out]
        n177 = property on="File Name" class="Str (strict)"() -> ("Value"=w265:T5)  [unwired: 2 in, 2 out]
        n178 = String Length(string=w265) -> (length=w264:i32)
        n179 = Equal To 0?(x=w264) -> (x = 0?=w263:bool)
        n180 = case shown="True" w263 {
          frame False {
          }
          frame True {
            n181 = One Button Dialog(message="A filename has not been entered!") -> ()  [unwired: 1 in, 1 out]
          }
        }
      }
      event "Stop Test Button": Value Change {
        n182 = event-data() -> ()  [unwired: 1 in, 5 out]
        n183 = flat-sequence {
          tunnel: w272 -> [w274]
          tunnel: [w274] -> w271
          tunnel: [w273] -> w269
          tunnel: w271 -> [w278]
          tunnel: [w277] -> w270
          tunnel: w269 -> [w277]
          tunnel: [w276] -> w268
          tunnel: w270 -> [w282]
          tunnel: w268 -> [w281]
          tunnel: [T11."Disabled and Grayed Out" ("Disabled")] -> w267
          frame #0 {
            n184 = local read "Connected?"() -> (w273:bool)
            n185 = local write "Stop Cmd"(T1 1.0 ("Stop Cmd")) -> ()
          }
          frame #1 {
            n186 = Enqueue Element(queue=w278, element=Control_3."main" ("Enum")) -> (queue out=w276:refnum<queue>)  [unwired: 2 in, 2 out]
          }
          frame #2 {
            n187 = case shown="True" w282 {
              tunnel: w281 -> [w283 w286]
              tunnel: [w283 w285] -> _
              frame False {
              }
              frame True {
                n188 = local write "Connected?"(FALSE ("Connected?")) -> ()
                n189 = Enqueue Element(queue=w286, element=Control_3."Multigas disconnect" ("Enum")) -> (queue out=w285:refnum<queue>)  [unwired: 2 in, 2 out]
              }
            }
          }
        }
        n190 = property on="Stop Test Button" class="Bool"("DisabledEnum"=w267) -> ()  [unwired: 2 in, 2 out]
      }
      event "Stopped?": Value Change {
        n191 = event-data() -> ()  [unwired: 1 in, 5 out]
        n192 = flat-sequence {
          tunnel: w290 -> [w294]
          tunnel: [w293] -> w289
          tunnel: [w292] -> w288
          tunnel: w289 -> [w296]
          tunnel: w288 -> [w295]
          frame #0 {
            n193 = local read "Connected?"() -> (w292:bool)
            n194 = Enqueue Element(queue=w294, element=Control_3."main" ("Enum")) -> (queue out=w293:refnum<queue>)  [unwired: 2 in, 2 out]
          }
          frame #1 {
            n195 = case shown="True" w295 {
              tunnel: w296 -> [_ w297]
              frame False {
              }
              frame True {
                n196 = local write "Connected?"(FALSE ("Connected?")) -> ()
                n197 = Enqueue Element(queue=w297, element=Control_3."Multigas disconnect" ("Enum")) -> ()  [unwired: 2 in, 3 out]
              }
            }
          }
        }
      }
      event "Alarm ack": Value Change {
        # "system alarm - set to off"
        n198 = event-data() -> ()  [unwired: 1 in, 5 out]
        n199 = local write "Acknowledge"(TRUE ("Acknowledge")) -> ()
        n200 = property on="Soft Alarm" class="Bool (strict)"("Value"=FALSE ("Acknowledge")) -> ()  [unwired: 2 in, 2 out]
        n201 = property on="Alarm ack" class="Bool"("DisabledEnum"=T11."Disabled and Grayed Out" ("Disabled")) -> ()  [unwired: 2 in, 2 out]
      }
      event "Purge System": Value Change {
        n202 = event-data() -> ()  [unwired: 1 in, 5 out]
        n203 = flat-sequence {
          tunnel: w304 -> [w306]
          tunnel: [w306] -> w303
          tunnel: w303 -> [w307]
          frame #0 {
            n204 = local write "Enum 1"(u16 4 ("Test number")) -> ()
          }
          frame #1 {
            n205 = Enqueue Element(queue=w307, element=Control_3."start test" ("Enum")) -> ()  [unwired: 2 in, 3 out]
          }
        }
      }
      event "Clear log": Value Change {
        n206 = event-data() -> ()  [unwired: 1 in, 5 out]
        n207 = local write "Table"(string[][] [] ("Table")) -> ()
      }
      event "Advanced settings": Value Change {
        # "To be updated"
        # "SO2 conc\nNOx conc\nCO conc\nHC conc\nBleed ratio N2\nBleed ratio CO2"
        n208 = event-data() -> ()  [unwired: 1 in, 5 out]
        n209 = call "Advanced settings MAX.vi"() -> ("output cluster"=→"output cluster":T2)  [unwired: 1 in]
      }
    }
    "stop 2" <- w39
  }
  n210 = node-c288(nitl_modes."Discard missed periods, maintain original phase" ("Mode")) -> (w9:T12)  [unwired: 4 in]
  n211 = node-c288() -> (w2:T12)  [unwired: 4 in]
  n212 = timed-loop {
    timing: w9 -> [_]
    timing-out: [_] -> w8
    shift-right: [w314] -> _
    shift-left: path "" -> [w456]
    shift-right: [w414] -> _
    shift-left: w3 -> [w455]
    shift-right: [w315] -> _
    shift-left: _ -> [w425]
    shift-right: [w404] -> _
    shift-left: w3 -> [w407]
    shift-right: [w405] -> _
    shift-left: w3 -> [w406]
    stop <- w454 stop-if-true
    w325 = 54321.0 ("y")
    # "0 Flow Rate 1\n1 Flow Rate 2\n2 CO2 U\n3 CO U\n4 HC U\n5 O2 U\n7 CO2 D\n8 CO D\n9 HC D\n10 O2 D\n12 TC1X\n13 TC2A\n14 TC3Y\n15 TC4B\n16 TC5\n17 TC6\n32 Venturi 1\n33 Venturi 2\n34 Tank\n35 Bearing 1\n36 Bearing 2\n38 Ex A\n39 Ex B\n40 Ex C\n41 Ex D\n42 Furnace 1\n43 Furnace 2\n44 NO 1 ?? \n45 Lambda 1\n46 NO 2 ??\n47 Lambda 2"
    # "ECM AFR"
    n213 = node-c288() -> (→"Finished Late? [i-1]":bool, →"Iteration Duration":i64)  [unwired: 1 in, 1 out]
    n214 = shared-variable "cRIO-9082\\Library 1.lvlib\\DATA"() -> (w453:dbl[])  [unwired: 1 in, 1 out]
    n215 = local read "MKS 1"() -> (w335:i16)
    n216 = local read "MKS 2"() -> (w334:i16)
    n217 = case shown="1" w334 {
      tunnel: [dbl[] [54321.0] w566] -> w331
      frame 0, Default {
      }
      frame 1 {
        # "Connecting to MKS Analyser 2"
        n218 = call "tw_PollRequest simple version.vi"("EVID list"=i32[] [2000, 2001, 2002, 2003, 2004, 2005, 2006, 2007, 2008, 2009, 2010, 2011, 2012, 2013, 2014], "IP_ADD [127.0.0.1]"="192.168.254.2") -> ("values out"=w564:string[])  [unwired: 7 in, 2 out]
        n219 = for {
          tunnel: [w568] -> w562 mode=indexing
          tunnel: w564 -> [w567] mode=indexing
          n220 = Fract/Exp String To Number(string=w567) -> (number=w568:dbl)  [unwired: 3 in, 1 out]
        }
        n221 = Build Array (concatenate)(w562) -> (w566:dbl[])
      }
    }
    n222 = case shown="1" w335 {
      tunnel: [dbl[] [54321.0] w570] -> w333
      frame 0, Default {
      }
      frame 1 {
        # "Connecting to MKS Analyser 1"
        n223 = call "tw_PollRequest simple version.vi"("EVID list"=i32[] [2000, 2001, 2002, 2003, 2004, 2005, 2006, 2007, 2008, 2009, 2010, 2011, 2012, 2013, 2014], "IP_ADD [127.0.0.1]"="192.168.254.1") -> ("values out"=w573:string[])  [unwired: 7 in, 2 out]
        n224 = for {
          tunnel: [w576] -> w571 mode=indexing
          tunnel: w573 -> [w575] mode=indexing
          n225 = Fract/Exp String To Number(string=w575) -> (number=w576:dbl)  [unwired: 3 in, 1 out]
        }
        n226 = Build Array (concatenate)(w571) -> (w570:dbl[])
      }
    }
    n227 = Type Cast(type=w453, x=w453) -> (*(type *) &x=w464:dbl[])
    n228 = local read "Advanced Logging"() -> (w320:bool)
    n229 = Delete From Array(array=w464, length=4, index=0) -> (deleted portion=w461:dbl[], array with subset deleted=w321:dbl[])
    n230 = local read "Full system?"() -> (w311:bool)
    n231 = case shown="False" w320 {
      tunnel: [w486 w537] -> w322
      tunnel: w321 -> [w487 w537]
      tunnel: [w485 "Time\tFlow 1 g/s\tFlow 2 g/s\tECM AFR\tCO2 U %\tCO U %\tHC U ppm\tO2 U %\tNO U ppm\tCO2 D %\tCO D %\tHC D ppm\tO2 D %\tNO D ppm\tTC1X\tTC2A\tTCY\tTC4B\tTC5\tTC6\tTC7\tTC8\tTC9\tTC10\tTC11\tTC12\tTC13\tTC14\tTC15\tTC16\tTC17\tTC18\tTC19\tTC20\tTC Vent 1\tTC Vent 2\tTC Tank\tTC Fan B1\tTC Fan B2\tTC Cab\tTC Ex A\tTC Ex B\tTC Ex C\tTC Ex D\tTC MFC Box\tTC Furn 1\tTC Furn 2\tTank Pressure\tRapidox\tLambda 1\tLambda 2\tNOX 1 ppm\tNOX 2 ppm\tUEGO 1\tUEGO 2" ("Heading string 2")] -> w319
      tunnel: w311 -> [w484 _]
      frame False {
        n232 = case shown="True" w484 {
          tunnel: w487 -> [w502 w517]
          tunnel: [w493 w519] -> w486
          tunnel: ["Time\tFlow 1 g/s\tCO2 U %\tCO U %\tHC U ppm\tO2 U %\tNO U ppm\tCO2 D %\tCO D %\tHC D ppm\tO2 D %\tNO D ppm\tTC1X\tTC2A\tTCY\tTC4B\tTC5\tTC6\tTC7\tTC8\tRapidox\tLambda 1\tLambda 2\tNOX 1 ppm\tNOX 2 ppm\tUEGO 1\tUEGO 2" ("Heading string 2") "Time\tFlow 1 g/s\tFlow 2 g/s\tCO2 U %\tCO U %\tHC U ppm\tO2 U %\tNO U ppm\tCO2 D %\tCO D %\tHC D ppm\tO2 D %\tNO D ppm\tTC1X\tTC2A\tTCY\tTC4B\tTC5\tTC6\tTC7\tTC8\tRapidox\tLambda 1\tLambda 2\tNOX 1 ppm\tNOX 2 ppm\tUEGO 1\tUEGO 2" ("Heading string 2")] -> w485
          frame False {
            n233 = Delete From Array(array=w502, length=21, index=0) -> (deleted portion=w489:dbl[], array with subset deleted=w501:dbl[])
            n234 = Index Array(array=w501, index #1=47 ("index"), index #2=48 ("index"), index #3=49 ("index"), index #4=50 ("index"), index #5=51 ("index"), index #6=52 ("index"), index #7=53 ("index")) -> (element #1=w500:dbl, element #2=w499:dbl, element #3=w498:dbl, element #4=w497:dbl, element #5=w496:dbl, element #6=w495:dbl, element #7=w494:dbl)
            n235 = Delete From Array(array=w489, length=1, index=2) -> (array with subset deleted=w488:dbl[])  [unwired: 1 out]
            n236 = Build Array (concatenate)(w488, w500, w499, w498, w497, w496, w495, w494) -> (w493:dbl[])
          }
          frame True {
            n237 = Delete From Array(array=w517, length=21, index=0) -> (deleted portion=w514:dbl[], array with subset deleted=w518:dbl[])
            n238 = Index Array(array=w518, index #1=47 ("index"), index #2=48 ("index"), index #3=49 ("index"), index #4=50 ("index"), index #5=51 ("index"), index #6=52 ("index"), index #7=53 ("index")) -> (element #1=w526:dbl, element #2=w525:dbl, element #3=w524:dbl, element #4=w523:dbl, element #5=w522:dbl, element #6=w521:dbl, element #7=w520:dbl)
            n239 = Delete From Array(array=w514, length=2, index=1) -> (array with subset deleted=w512:dbl[])  [unwired: 1 out]
            n240 = Build Array (concatenate)(w512, w526, w525, w524, w523, w522, w521, w520) -> (w519:dbl[])
          }
        }
      }
      frame True {
        (unwired) "Time\tFlow 1 g/s\tFlow 2 g/s\tECM AFR\tCO2 U %\tCO U %\tHC U ppm\tO2 U %\tNO U ppm\tCO2 D %\tCO D %\tHC D ppm\tO2 D %\tNO D ppm\tTC1X\tTC2A\tTCY\tTC4B\tTC5\tTC6\tTC7\tTC8\tTC9\tTC10\tTC11\tTC12\tTC13\tTC14\tTC15\tTC16\tTC17\tTC18\tTC19\tTC20\tTC Vent 1\tTC Vent 2\tTC Fan B1\tTC Fan B2\tTC Cab\tTC Ex A\tTC Ex B\tTC Ex C\tTC Ex D\tTC Furn 1\tTC Furn 2\tNOX 1 ppm\tNLambda 1\tNOX 2 ppm\tNLambda 2\tEGO 1\tEGO 2\tEGO 3\tEGO 4\tCO2 U %\tCO U %\tHC U ppm\tO2 U %\tNO U ppm\tCO2 D %\tCO D %\tHC D ppm\tO2 D %\tNO D ppm\r\n" ("Heading string 2")
      }
    }
    n241 = Index Array(array=w461) -> (element #1=w315:dbl, element #2=w431:dbl, element #3=w317:dbl, element #4=w424:dbl)  [unwired: 4 in]
    "Error" <- w317
    n242 = To Unsigned Long Integer(number=w424) -> (unsigned 32bit integer=w423:u32)
    n243 = Number To Boolean Array(number=w423) -> (Boolean array=w443:bool[])
    n244 = Index Array(array=w443) -> (element #2=w441:bool, element #3=w440:bool, element #4=w420:bool)  [unwired: 4 in, 1 out]
    "Extractor Fan On" <- w420
    n245 = case shown="2" w431 {
      tunnel: [w596 TRUE FALSE] -> w430
      tunnel: [w597 FALSE TRUE] -> w429
      frame 0, Default {
        n246 = local read "Pass"() -> (w597:bool)
        n247 = local read "Fail"() -> (w596:bool)
      }
      frame 1 {
      }
      frame 2 {
      }
    }
    "Pass" <- w429
    "Fail" <- w430
    n248 = Or(x=w441, y=w440) -> (x .or. y?=→"Doors Open":bool)
    n249 = Not(x=w420) -> (.not. x?=→"Doors Unlocked":bool)
    n250 = Less?(x=w315, y=w425) -> (x < y?=w422:bool)
    n251 = Path To String(path="File Path") -> (string=w418:string)
    n252 = Index Array(array=w333, index=0) -> (element=w329:dbl)
    n253 = Index Array(array=w331, index=0) -> (element=w327:dbl)
    n254 = local read "Connected"() -> (w421:bool)
    n255 = Concatenate Strings(w418, "\\" ("string"), "File Name") -> (w336:string)
    n256 = Not Equal?(x=w329, y=w325) -> (x != y?=w328:bool)
    n257 = Not Equal?(x=w325, y=w327) -> (x != y?=w326:bool)
    n258 = case shown="False" w328 {
      tunnel: [w543 w554] -> w324
      tunnel: w331 -> [w542 w553]
      tunnel: w333 -> [_ w552]
      tunnel: w326 -> [w541 w551]
      tunnel: [w540 w548] -> w323
      frame False {
        n259 = case shown="False" w541 {
          tunnel: [dbl[] [54321.0] w547] -> w543
          tunnel: w542 -> [_ w547]
          tunnel: ["\r\n" ("Heading string 2") "\tNO\tNO2 (150)\tNO2 (2000)\tN2O\tNH3 (300)\tNH3 (3000)\tHNCO (400)\tH2O\tCO2\tCO (500)\tCO (1)\tCH4 (250)\tCH4 (3000)\tNOxP\tPropane\r\n" ("Heading string 2")] -> w538
          frame False {
          }
          frame True {
          }
        }
        n260 = Build Array(" " ("Heading string 2"), w538) -> (w540:string[])
      }
      frame True {
        n261 = case shown="True" w551 {
          tunnel: [w556 w560] -> w554
          tunnel: w553 -> [_ w559]
          tunnel: w552 -> [w556 w558]
          tunnel: ["\rn" ("Heading string 2") "\tNO\tNO2 (150)\tNO2 (2000)\tN2O\tNH3 (300)\tNH3 (3000)\tHNCO (400)\tH2O\tCO2\tCO (500)\tCO (1)\tCH4 (250)\tCH4 (3000)\tNOxP\tPropane\r" ("Heading string 2")] -> w549
          frame False {
          }
          frame True {
            n262 = Build Array (concatenate)(w558, w559) -> (w560:dbl[])
          }
        }
        n263 = Build Array("\tNO\tNO2 (150)\tNO2 (2000)\tN2O\tNH3 (300)\tNH3 (3000)\tHNCO (400)\tH2O\tCO2\tCO (500)\tCO (1)\tCH4 (250)\tCH4 (3000)\tNOxP\tPropane" ("Heading string 2"), w549) -> (w548:string[])
      }
    }
    n264 = And(x=w421, y=w422) -> (x .and. y?=w413:bool)
    n265 = local write "Stopped?"(w413) -> ()
    n266 = Equal To 0?(x=w317) -> (x = 0?=w318:bool)
    n267 = Equal To 0?(x=w315) -> (x = 0?=w316:bool)
    n268 = Build Array (concatenate)(w322, w324) -> (w457:dbl[])
    n269 = Equal?(x=w315, y=2.0) -> (x = y?=w349:bool)
    n270 = String To Path(string=w336) -> (path=w415:path)
    n271 = Build Array(w318, w316) -> (w437:bool[])
    n272 = Equal?(x=w315, y=3.0) -> (x = y?=w341:bool)
    n273 = Equal?(x=w315, y=4.0) -> (x = y?=w339:bool)
    n274 = Boolean Array To Number(Boolean array=w437) -> (number=w436:u32)
    n275 = Not Equal?(x=w415, y=w456) -> (x != y?=w466:bool)
    n276 = Compound Arithmetic op=OR(w349, w341, w339) -> (w348:bool)
    n277 = local read "Log Test Button"() -> (w337:bool)
    n278 = case shown="0, Default" w436 {
      tunnel: [w621 w622 w627 w629] -> w438
      tunnel: [w621 w622 w627 w629] -> w435
      tunnel: [w621 w622 w627 w629] -> w434
      tunnel: [w621 w622 w625 w629] -> w433
      tunnel: [T11."Enabled" ("Disabled") T11."Enabled" ("Disabled") w625 w629] -> w432
      tunnel: [FALSE FALSE FALSE TRUE] -> w412
      frame 0, Default {
        w621 = T11."Disabled and Grayed Out" ("Disabled")
      }
      frame 1 {
        w622 = T11."Disabled and Grayed Out" ("Disabled")
      }
      frame 2 {
        w625 = T11."Enabled" ("Disabled")
        w627 = T11."Disabled and Grayed Out" ("Disabled")
      }
      frame 3 {
        w629 = T11."Enabled" ("Disabled")
        (unwired) T11."Disabled and Grayed Out" ("Disabled")
      }
    }
    n279 = for {
      tunnel: w457 -> [w637] mode=indexing
      tunnel: [w636] -> w468 mode=indexing
      n280 = Number To Fractional String(number=w637, precision (6)=i16 3) -> (F-format string=w636:string)  [unwired: 2 in]
    }
    n281 = Select(t=w415, s=w466, f=w456) -> (s? t:f=w467:path)
    n282 = case shown="True" w466 {
      tunnel: w467 -> [w630 w635]
      tunnel: [w630 w634] -> w465
      tunnel: w323 -> [_ w632]
      tunnel: w319 -> [_ w631]
      frame False {
      }
      frame True {
        # "setting up the header"
        n283 = Build Array (concatenate)(w631, w632) -> (w633:string[])
        n284 = call-poly <vilib>:"Write To Spreadsheet File.vi"("1D data"=w633, "file path (dialog if empty)"=w635) -> ("new file path (Not A Path if cancelled)"=w634:path)  [unwired: 6 in]
      }
    }
    n285 = And(x=w337, y=w348) -> (x .and. y?=w483:bool)
    "Log?" <- w483
    n286 = Equal?(x=w315, y=0.0) -> (x = y?=w401:bool)
    n287 = case shown="5" w315 {
      tunnel: [w583 w586 w588 w590 TRUE FALSE] -> w428
      tunnel: [w583 TRUE TRUE TRUE w592 w594] -> w427
      tunnel: [TRUE w586 w588 w590 w592 w594] -> w426
      frame 0, Default {
        w583 = FALSE
      }
      frame 1 {
        w586 = FALSE
      }
      frame 2 {
        w588 = FALSE
      }
      frame 3 {
        w590 = FALSE
      }
      frame 4 {
        w592 = FALSE
        n288 = local write "Stop Cmd"(T1 0.0 ("Stop Cmd")) -> ()
      }
      frame 5 {
        w594 = FALSE
      }
    }
    "Cool Down" <- w428
    "Test In Progress" <- w427
    "Standby" <- w426
    n289 = property on="Start Test Button" class="Bool"("DisabledEnum"=w438) -> ()  [unwired: 2 in, 2 out]
    n290 = property on="Execute Leak Test Button" class="Bool"("DisabledEnum"=w435) -> ()  [unwired: 2 in, 2 out]
    n291 = property on="Compile Test Button" class="Bool"("DisabledEnum"=w434) -> ()  [unwired: 2 in, 2 out]
    n292 = property on="Purge System" class="Bool"("DisabledEnum"=w433) -> ()  [unwired: 2 in, 2 out]
    n293 = property on="Advanced settings" class="Bool"("DisabledEnum"=w432) -> ()  [unwired: 2 in, 2 out]
    n294 = property class="VI"("Front Panel.Closeable"=w412) -> ()  [unwired: 2 in, 2 out]
    n295 = Delete From Array(array=w321, length=1, index=2) -> (deleted portion=w345:dbl[], array with subset deleted=w343:dbl[])
    n296 = Index Array(array=w324, index #1=0 ("index"), index #2=1 ("index"), index #3=2 ("index"), index #4=3 ("index")) -> ()  [unwired: 4 out]
    n297 = Index Array(array=w345) -> (element=w344:dbl)  [unwired: 1 in]
    n298 = local read "Full system?"() -> (w402:bool)
    n299 = Not Equal To 0?(x=w317) -> (x != 0?=w459:bool)
    n300 = Not Equal?(x=w317, y=w455) -> (x != y?=w458:bool)
    n301 = case shown="True" w483 {
      tunnel: w465 -> [w641 w649]
      tunnel: [w641 w661] -> w314
      tunnel: w468 -> [_ w657]
      tunnel: w407 -> [_ w650]
      tunnel: w406 -> [w640 w645]
      tunnel: [w640 w647] -> w405
      tunnel: [w639 w646] -> w404
      frame False {
        n302 = local read "Log interval (seconds)"() -> (w639:T1)
      }
      frame True {
        n303 = Get Date/Time In Seconds() -> (seconds since 1Jan1904=w658:timestamp)
        n304 = Decrement(x=w650) -> (x-1=w651:T1)
        n305 = Less Than 0?(x=w651) -> (x < 0?=w652:bool)
        n306 = Equal To 0?(x=w651) -> (x = 0?=w653:bool)
        n307 = Build Array(w652, w653) -> (w654:bool[])
        n308 = Path To String(path=w649) -> (string=w644:string)
        "File name" <- w644
        n309 = Format Date/Time String(time format string (%c)="%d/%m/%y %H:%M:%S", seconds (now)=w658) -> (date/time string=w659:string)  [unwired: 1 in]
        n310 = Boolean Array To Number(Boolean array=w654) -> (number=w655:u32)
        n311 = case shown="2" w655 {
          tunnel: w650 -> [w668 w669 _]
          tunnel: [w667 w669 w672] -> w646
          tunnel: w644 -> [w666 w671 w675]
          tunnel: [w663 w671 w673] -> w648
          tunnel: [w662 w670 w674] -> w647
          tunnel: w645 -> [w662 w670 w678]
          frame 0, Default {
            n312 = Number To Decimal String(number=w662) -> (decimal integer string=w664:string)  [unwired: 1 in]
            n313 = call <vilib>:"Space Constant.vi"() -> ("String"=w665:string)
            n314 = Decrement(x=w668) -> (x-1=w667:T1)
            n315 = Concatenate Strings(w666, w665, w664) -> (w663:string)
          }
          frame 1 {
          }
          frame 2 {
            n316 = Increment(x=w678) -> (x+1=w674:dbl)
            n317 = local read "Log interval (seconds)"() -> (w672:T1)
            n318 = Number To Decimal String(number=w674) -> (decimal integer string=w676:string)  [unwired: 1 in]
            n319 = call <vilib>:"Space Constant.vi"() -> ("String"=w677:string)
            n320 = Concatenate Strings(w675, w677, w676) -> (w673:string)
          }
        }
        n321 = Build Array (concatenate)(w659, w657) -> (w643:string[])
        n322 = String To Path(string=w648) -> (path=w642:path)
        n323 = call-poly <vilib>:"Write To Spreadsheet File.vi"("append to file? (new file:F)"=TRUE, "1D data"=w643, "file path (dialog if empty)"=w642) -> ("new file path (Not A Path if cancelled)"=w661:path)  [unwired: 5 in]
      }
    }
    n324 = And(x=w459, y=w458) -> (x .and. y?=w460:bool)
    n325 = Index Array(array=w343, index #1=0 ("index"), index #2=1 ("index"), index #3=2 ("index"), index #4=3 ("index"), index #5=4 ("index"), index #6=5 ("index"), index #7=7 ("index"), index #8=8 ("index"), index #9=9 ("index"), index #10=10 ("index"), index #11=12 ("index"), index #12=13 ("index"), index #13=14 ("index"), index #14=15 ("index"), index #15=16 ("index"), index #16=17 ("index"), index #17=32 ("index"), index #18=33 ("index"), index #19=34 ("index"), index #20=35 ("index"), index #21=36 ("index"), index #22=38 ("index"), index #23=39 ("index"), index #24=40 ("index"), index #25=41 ("index"), index #26=43 ("index"), index #27=44 ("index"), index #28=49 ("index"), index #29=50 ("index"), index #30=47 ("index"), index #31=48 ("index")) -> (element #1=w399:dbl, element #2=w398:dbl, element #3=w395:dbl, element #4=w393:dbl, element #5=w394:dbl, element #6=w392:dbl, element #7=w391:dbl, element #8=w390:dbl, element #9=w389:dbl, element #10=w388:dbl, element #11=w383:dbl, element #12=w382:dbl, element #13=w381:dbl, element #14=w380:dbl, element #15=w379:dbl, element #16=w378:dbl, element #17=w372:dbl, element #18=w371:dbl, element #19=w370:dbl, element #20=w369:dbl, element #21=w368:dbl, element #22=w363:dbl, element #23=w362:dbl, element #24=w361:dbl, element #25=w360:dbl, element #26=→"Furnace temp 1":dbl, element #27=→"Furnace temp 2":dbl, element #28=w353:dbl, element #29=w313:dbl, element #30=w312:dbl, element #31=w350:dbl)
    n326 = Build Array(w402, w401) -> (w403:bool[])
    n327 = case shown="True" w460 {
      tunnel: w317 -> [w603 w614]
      tunnel: w458 -> [w606 _]
      tunnel: [w602 w614] -> w414
      frame False {
        n328 = Equal To 0?(x=w603) -> (x = 0?=w607:bool)
        n329 = And(x=w607, y=w606) -> (x .and. y?=w605:bool)
        n330 = case shown="True" w605 {
          frame False {
          }
          frame True {
            w610 = FALSE ("Ack hard alarm!")
            n331 = property on="Hard Alarm" class="Bool (strict)"("Value"=w610) -> ()  [unwired: 2 in, 2 out]
            n332 = property on="System Alarm" class="Bool (strict)"("Value"=w610) -> ()  [unwired: 2 in, 2 out]
          }
        }
        n333 = case shown="False" "Acknowledge" {
          tunnel: [w608 0.0 ("Numeric")] -> w602
          tunnel: w603 -> [w608 _]
          frame False {
          }
          frame True {
          }
        }
      }
      frame True {
        n334 = local read "Table"() -> (w617:string[][])
        n335 = call "Error list.vi"("Error code"=w614, "Error array in"=w617) -> ("Hard alarm?"=w611:bool, "Error array out"=w616:string[][])  [unwired: 8 in]
        "Hard Alarm" <- w611
        "System Alarm" <- w611
        n336 = Not(x=w611) -> (.not. x?=w612:bool)
        "Soft Alarm" <- w612
        n337 = case shown="True" w612 {
          frame False {
          }
          frame True {
            n338 = property on="Alarm ack" class="Bool"("DisabledEnum"=T11."Enabled" ("Disabled")) -> ()  [unwired: 2 in, 2 out]
          }
        }
        n339 = local write "Table"(w616) -> ()
        n340 = local write "Acknowledge"(FALSE ("Acknowledge")) -> ()
        n341 = property on="Tab Control" class="TabCtl (strict)"("Value"=6) -> ()  [unwired: 2 in, 2 out]
      }
    }
    n342 = Boolean Array To Number(Boolean array=w403) -> (number=w400:u32)
    n343 = case shown="1" w400 {
      tunnel: w399 -> [w578 w580 _ _]
      tunnel: w398 -> [_ w579 _ _]
      tunnel: [w578 w580 w581 w582] -> w397
      tunnel: [0.0 ("y") w579 w581 w582] -> w396
      frame 0, Default {
      }
      frame 1 {
      }
      frame 2 {
        w581 = 0.0 ("y")
      }
      frame 3 {
        w582 = 0.0 ("y")
      }
    }
    n344 = Merge Signals(w397, w396) -> (→"Flow Rate (g/s)":dynamicdata)
    n345 = Merge Signals(w395, w393, w392, w391, w390, w388) -> (→"M584L Upstream & Downstream":dynamicdata)
    n346 = Merge Signals(w394, w389) -> (→"HC Concentration (ppm)":dynamicdata)
    n347 = Merge Signals(w383, w382, w381, w380, w379, w378) -> (→"Sample Temperatures (°C)":dynamicdata)
    n348 = Merge Signals(w372, w371, w370, w369, w368) -> (→"System Temperatures (°C)":dynamicdata)
    n349 = Merge Signals(w363, w362, w361, w360) -> (→"Heat Exchanger Temperatures (°C)":dynamicdata)
    n350 = Merge Signals(w353, w313) -> (→"NO Concentration (ppm)":dynamicdata)
    n351 = Merge Signals(w312, w350, w344) -> (→"Lambda":dynamicdata)
    n352 = local read "stop 2"() -> (w454:bool)
    n353 = node-c288() -> ()  [unwired: 1 in, 1 out]
  }
  n354 = timed-loop {
    timing: w2 -> [_]
    timing-out: [_] -> w1
    stop <- _ stop-if-true
    n355 = node-c288() -> ()  [unwired: 1 in, 1 out]
    n356 = shared-variable "cRIO-9082\\Library 1.lvlib\\DATA_2"() -> (w693:dbl[])  [unwired: 1 in, 1 out]
    n357 = for {
      tunnel: w693 -> [w700] mode=indexing
      tunnel: [w699] -> w685 mode=indexing
      n358 = Number To Fractional String(number=w700, precision (6)=i16 3) -> (F-format string=w699:string)  [unwired: 2 in]
    }
    n359 = Get Date/Time In Seconds() -> (seconds since 1Jan1904=w688:timestamp)
    n360 = local read "File name"() -> (w692:string)
    n361 = Format Date/Time String(time format string (%c)="%d/%m/%y %H:%M:%S", seconds (now)=w688) -> (date/time string=w686:string)  [unwired: 1 in]
    n362 = Concatenate Strings(w692, "_MFC" ("string")) -> (w690:string)
    n363 = Build Array (concatenate)(w686, w685) -> (w684:string[])
    n364 = String To Path(string=w690) -> (path=w687:path)
    n365 = local read "Log?"() -> (w683:bool)
    n366 = case shown="True" w683 {
      tunnel: w687 -> [w694 w697]
      tunnel: [w694 w695] -> _
      tunnel: w684 -> [_ w696]
      frame False {
      }
      frame True {
        n367 = call-poly <vilib>:"Write To Spreadsheet File.vi"("append to file? (new file:F)"=TRUE, "1D data"=w696, "file path (dialog if empty)"=w697) -> ("new file path (Not A Path if cancelled)"=w695:path)  [unwired: 5 in]
      }
    }
    n368 = node-c288() -> ()  [unwired: 1 in, 1 out]
  }
  n369 = while {
    tunnel: w37 -> [w708]
    tunnel: w21 -> [w706]
    tunnel: w23 -> [w705]
    tunnel: [FALSE ("stop 2")] -> w11
    stop <- w709 stop-if-true
    n370 = Dequeue Element(queue=w708) -> (element=w707:T10)  [unwired: 2 in, 3 out]
    n371 = case shown="\"main\", Default" w707 {
      tunnel: w706 -> [_ _ _ w760 w771 w807 w841 _ _ _ _ _ _ _ w1204 _ _ _ _ _ _ _]
      tunnel: w705 -> [_ _ _ _ _ _ _ _ w854 w869 w924 w969 _ _ _ _ _ _ _ _ _ _]
      frame "main", Default {
        # "20"
        # "25"
        # "30"
        # "15"
        # "10"
        # "5"
        # "0"
        # "30"
        # "25"
        # "20"
        # "15"
        # "10"
        # "5"
        # "0"
        # "Output Cluster\n\n0 NOx Conc\n1 CO conc %\n2 HC conc %\n3 Bleed H2O \n4 Bleed CO2\n5 Bleed N2 \n6 lambda P\n7 lambda I\n8 lambda D\n9 purge duration\n10 Target furnace lambda\n11 HC reaction ct\n12 Full system\n13 Log interval\n14 MKS 1\n15 MKS 2"
        n372 = local read "output cluster"() -> (w734:T2)
        n373 = Unbundle(w734) -> ("NOx Concentration (ppm)"=w720:T1, "CO concentration %"=w719:T1, "HC concentration %"=w718:T1, "Bleed H2O %"=w717:T1, "Bleed CO2 %"=w716:T1, "Bleed N2 %"=w731:T1, "lambda P"=w730:T1, "lambda I"=w729:T1, "lambda D"=w732:T1, "Purge duration (seconds)"=w733:T1, "Target furnace lambda"=w725:T1, "HC reaction constant"=w724:T1, w726:i16, "Log interval (HRS)"=→"Log interval (seconds)":T1, w713:i16, w711:i16, "Advanced Logging"=→"Advanced Logging":bool)
        "MKS 1" <- w713
        "MKS 2" <- w711
        n374 = local read "Test Flow Rate(g/s)"() -> (w746:T1)
        n375 = local read "Test number"() -> (w751:u16)
        n376 = local read "Inlet LAMBDA"() -> (w738:T1)
        n377 = local read "NO ppm Loff"() -> (w736:T1)
        n378 = local read "NO:CO Ratio"() -> (w735:T1)
        n379 = local read "Inlet O2 (%)"() -> (w737:T1)
        n380 = local read "Connected"() -> (w740:bool)
        n381 = Boolean To (0,1)(Boolean=w740) -> (0, 1=w723:i16)
        n382 = Not Equal To 0?(x=w713) -> (x != 0?=w714:bool)
        n383 = Not Equal To 0?(x=w711) -> (x != 0?=w712:bool)
        n384 = Or(x=w714, y=w712) -> (x .or. y?=→"Connected":bool)
        n385 = Not Equal To 0?(x=w726) -> (x != 0?=→"Full system?":bool)
        n386 = Build Array("Stop Cmd", w751, w746, "Test Start Temperature (°C)", "Test Stop temperature (°C)", "Furnace Ramp Rate (°C/min)", w738, w737, "Inlet LAMBDA Rich", "Inlet LAMBDA Lean", "Inlet Temperature (°C)", "NO ppm SW", w736, w735, "Temperature Limit (°C)", w723, "Inlet temp Age", "Flow rate Age", w720, w719, w718, w717, w716, w731, w730, w729, w732, w733, w725, w724, w726) -> (w742:T1[])
        n387 = shared-variable "cRIO-9082\\Library 1.lvlib\\Control Variables"(w742) -> ()  [unwired: 1 in, 1 out]
      }
      frame "start test" {
        w752 = FALSE
        n388 = property on="Pass" class="Bool (strict)"("Value"=w752) -> ()  [unwired: 2 in, 2 out]
        n389 = property on="Fail" class="Bool (strict)"("Value"=w752) -> ()  [unwired: 2 in, 2 out]
        n390 = local write "Pass"(w752) -> ()
        n391 = local write "Fail"(w752) -> ()
        n392 = shared-variable "cRIO-9082\\Library 1.lvlib\\Enum 1"("Enum 1") -> ()  [unwired: 1 in, 1 out]
      }
      frame "clear table 1" {
        n393 = property on="Sub-Cycle Name" class="Str (strict)"("Value"="" ("Subcycle name")) -> ()  [unwired: 2 in, 2 out]
        n394 = local write "Flag1"(FALSE) -> ()
        n395 = local write "Sub-Cycle Pattern"(string[][] [["", "0", "", "", "", "", "", "", "", "", "", "", ""], ["", "", "", "", "", "", "", "", "", "", "", "", ""], ["", "", "", "", "", "", "", "", "", "", "", "", ""], ["", "", "", "", "", "", "", "", "", "", "", "", ""], ["", "", "", "", "", "", "", "", "", "", "", "", ""], ["", "", "", "", "", "", "", "", "", "", "", "", ""], ["", "", "", "", "", "", "", "", "", "", "", "", ""], ["", "", "", "", "", "", "", "", "", "", "", "", ""], ["", "", "", "", "", "", "", "", "", "", "", "", ""], ["", "", "", "", "", "", "", "", "", "", "", "", ""], ["", "", "", "", "", "", "", "", "", "", "", "", ""], ["", "", "", "", "", "", "", "", "", "", "", "", ""], ["", "", "", "", "", "", "", "", "", "", "", "", ""], ["", "", "", "", "", "", "", "", "", "", "", "", ""], ["", "", "", "", "", "", "", "", "", "", "", "", ""], ["", "", "", "", "", "", "", "", "", "", "", "", ""], ["", "", "", "", "", "", "", "", "", "", "", "", ""], ["", "", "", "", "", "", "", "", "", "", "", "", ""], ["", "", "", "", "", "", "", "", "", "", "", "", ""], ["", "", "", "", "", "", "", "", "", "", "", "", ""], ["", "", "", "", "", "", "", "", "", "", "", "", ""], ["", "", "", "", "", "", "", "", "", "", "", "", ""], ["", "", "", "", "", "", "", "", "", "", "", "", ""], ["", "", "", "", "", "", "", "", "", "", "", "", ""], ["", "", "", "", "", "", "", "", "", "", "", "", ""], ["", "", "", "", "", "", "", "", "", "", "", "", ""], ["", "", "", "", "", "", "", "", "", "", "", "", ""], ["", "", "", "", "", "", "", "", "", "", "", "", ""], ["", "", "", "", "", "", "", "", "", "", "", "", ""], ["", "", "", "", "", "", "", "", "", "", "", "", ""], ["", "", "", "", "", "", "", "", "", "", "", "", ""]]) -> ()
      }
      frame "update list 1" {
        n396 = String To Path(string=w760) -> (path=w759:path)
        n397 = List Folder(path=w759, pattern="*.eyes") -> (filenames=w758:string[])  [unwired: 2 in, 3 out]
        n398 = property on="Sub-Cycle List" class="LstBox (strict)"("Item Names"=w758) -> ()  [unwired: 2 in, 2 out]
      }
      frame "save subc" {
        w764 = ".eyes" ("string")
        n399 = local read "Sub-Cycle Name"() -> (w763:T5)
        n400 = String To Path(string=w771) -> (path=w776:path)
        n401 = Equal?(x=w763, y="") -> (x = y?=w768:bool)
        n402 = List Folder(path=w776, pattern="*.eyes" ("string")) -> (filenames=w775:string[])  [unwired: 2 in, 3 out]
        n403 = Concatenate Strings(w763, w764) -> (w762:string)
        n404 = Concatenate Strings(w771, w763, w764) -> (w777:string)
        n405 = Search 1D Array(1D array=w775, element=w762) -> (index of element=w774:i32)  [unwired: 1 in]
        n406 = case shown="True" w768 {
          tunnel: [TRUE FALSE] -> w767
          frame False {
          }
          frame True {
            n407 = One Button Dialog(message="Insert file name!") -> ()  [unwired: 1 in, 1 out]
          }
        }
        n408 = String To Path(string=w777) -> (path=w770:path)
        n409 = Equal?(x=w774, y=-1) -> (x = y?=w772:bool)
        n410 = case shown="False" w772 {
          selector: w772 -> [_ w783]
          tunnel: [w781 w783] -> w766
          frame False {
            n411 = Two Button Dialog(message="A file with this name already exists!\nDo you want to overwrite?") -> (T button?=w781:bool)  [unwired: 2 in]
          }
          frame True {
          }
        }
        n412 = And(x=w766, y=w767) -> (x .and. y?=w765:bool)
        n413 = case shown="True" w765 {
          tunnel: w770 -> [_ w788]
          frame False {
          }
          frame True {
            n414 = local read "Sub-Cycle Pattern"() -> (w787:string[][])
            n415 = call "Table check.vi"("Input table"=w787) -> ("Incomplete?"=w785:bool, "Length"=w786:i32)  [unwired: 9 in]
            n416 = case shown="False" w785 {
              tunnel: w787 -> [w796 _]
              tunnel: w788 -> [w795 _]
              tunnel: w786 -> [w794 _]
              tunnel: string[] [] -> [w793 _]
              frame False {
                n417 = for {
                  N: w794 -> [_]
                  tunnel: w796 -> [w803]
                  shift-right: [w800] -> w792
                  shift-left: w793 -> [w801]
                  i -> [w802]
                  n418 = Index Array(array=w803, index (row)=w802) -> (element=w799:string[])  [unwired: 1 in]
                  n419 = Delete From Array(array=w799, index=0) -> (array with subset deleted=w798:string[])  [unwired: 1 in, 1 out]
                  n420 = Build Array (concatenate)(w801, w798) -> (w800:string[])
                }
                n421 = Build Array (concatenate)("SubCycle Data File for EYECAT - do not modify", w792) -> (w790:string[])
                n422 = call-poly <vilib>:"Write To Spreadsheet File.vi"("1D data"=w790, "file path (dialog if empty)"=w795) -> ()  [unwired: 6 in, 1 out]
              }
              frame True {
                n423 = One Button Dialog(message="The table is incomplete!\nplease review and save again!") -> ()  [unwired: 1 in, 1 out]
              }
            }
            n424 = local write "Flag1"(FALSE) -> ()
          }
        }
      }
      frame "load subc" {
        n425 = local read "Flag1"() -> (w808:bool)
        n426 = case shown="True" w808 {
          tunnel: [w835 w837] -> w806
          tunnel: w807 -> [w835 w837]
          tunnel: [TRUE w836] -> w805
          frame False {
          }
          frame True {
            n427 = Two Button Dialog(message="The table has been modified.\nDo you want to continue?") -> (T button?=w836:bool)  [unwired: 2 in]
          }
        }
        n428 = case shown="True" w805 {
          tunnel: w806 -> [_ w812]
          frame False {
          }
          frame True {
            n429 = property on="Sub-Cycle List" class="LstBox (strict)"() -> ("Item Names"=w824:string[])  [unwired: 2 in, 2 out]
            n430 = Index Array(array=w824, index="Sub-Cycle List") -> (element=w811:string)
            n431 = Concatenate Strings(w812, w811) -> (w822:string)
            n432 = Search/Split String(string=w811, search string/char (-)=".") -> (substring before match=w809:string)  [unwired: 1 in, 2 out]
            n433 = local write "Sub-Cycle Name"(w809) -> ()
            n434 = String To Path(string=w822) -> (path=w821:path)
            n435 = call-poly <vilib>:"Read From Spreadsheet File.vi"("file path (dialog if empty)"=w821) -> ("first row"=w817:string[])  [unwired: 6 in, 4 out]
            n436 = Delete From Array(array=w817, length=1, index=0) -> (array with subset deleted=w814:string[])  [unwired: 1 out]
            n437 = Array Size(array=w814) -> (size(s)=w820:i32)
            n438 = Divide(x=w820, y=12) -> (x/y=w813:dbl)
            n439 = for {
              N: w813 -> [_]
              shift-right: [w830] -> _
              shift-left: w814 -> [w833]
              tunnel: [w829] -> w818 mode=indexing
              i -> [w828]
              n440 = Increment(x=w828) -> (x+1=w827:i32)
              n441 = Delete From Array(array=w833, length=12, index=0) -> (deleted portion=w825:string[], array with subset deleted=w830:string[])
              n442 = Number To Decimal String(number=w827) -> (decimal integer string=w826:string)  [unwired: 1 in]
              n443 = Build Array (concatenate)(w826, w825) -> (w829:string[])
            }
            n444 = local write "Sub-Cycle Pattern"(w818) -> ()
          }
        }
      }
      frame "delete subc" {
        n445 = Two Button Dialog(message="This operation will permanently delete this file!\nDo you want to continue?") -> (T button?=w840:bool)  [unwired: 2 in]
        n446 = case shown="True" w840 {
          tunnel: w841 -> [_ w846]
          frame False {
          }
          frame True {
            n447 = local read "Sub-Cycle List"() -> (w843:i32)
            n448 = property on="Sub-Cycle List" class="LstBox (strict)"() -> ("Item Names"=w844:string[])  [unwired: 2 in, 2 out]
            n449 = Index Array(array=w844, index=w843) -> (element=w848:string)
            n450 = Concatenate Strings(w846, w848) -> (w847:string)
            n451 = local write "Flag1"(FALSE) -> ()
            n452 = String To Path(string=w847) -> (path=w845:path)
            n453 = Delete(path (use dialog)=w845) -> ()  [unwired: 4 in, 3 out]
          }
        }
      }
      frame "clear table 2" {
        n454 = property on="Cycle Name" class="Str (strict)"("Value"="" ("Subcycle name")) -> ()  [unwired: 2 in, 2 out]
        n455 = local write "Flag 2"(FALSE) -> ()
        n456 = local write "Cycle Pattern"(string[][] [["", "", "", "", ""], ["", "", "", "", ""], ["", "", "", "", ""], ["", "", "", "", ""], ["", "", "", "", ""], ["", "", "", "", ""], ["", "", "", "", ""], ["", "", "", "", ""], ["", "", "", "", ""], ["", "", "", "", ""], ["", "", "", "", ""], ["", "", "", "", ""], ["", "", "", "", ""], ["", "", "", "", ""], ["", "", "", "", ""], ["", "", "", "", ""], ["", "", "", "", ""], ["", "", "", "", ""], ["", "", "", "", ""], ["", "", "", "", ""], ["", "", "", "", ""], ["", "", "", "", ""], ["", "", "", "", ""], ["", "", "", "", ""], ["", "", "", "", ""], ["", "", "", "", ""], ["", "", "", "", ""], ["", "", "", "", ""], ["", "", "", "", ""], ["", "", "", "", ""], ["", "", "", "", ""]]) -> ()
      }
      frame "update list 2" {
        n457 = String To Path(string=w854) -> (path=w855:path)
        n458 = List Folder(path=w855, pattern="*.eyec") -> (filenames=w853:string[])  [unwired: 2 in, 3 out]
        n459 = property on="Cycle List" class="LstBox (strict)"("Item Names"=w853) -> ()  [unwired: 2 in, 2 out]
      }
      frame "save cycle" {
        w856 = ".eyec" ("string")
        n460 = local read "Cycle Name"() -> (w857:T5)
        n461 = String To Path(string=w869) -> (path=w870:path)
        n462 = List Folder(path=w870, pattern="*.eyec" ("string")) -> (filenames=w868:string[])  [unwired: 2 in, 3 out]
        n463 = Equal?(x=w857, y="") -> (x = y?=w863:bool)
        n464 = Concatenate Strings(w857, w856) -> (w859:string)
        n465 = Search 1D Array(1D array=w868, element=w859) -> (index of element=w867:i32)  [unwired: 1 in]
        n466 = Concatenate Strings(w869, w857, w856) -> (w872:string)
        n467 = case shown="True" w863 {
          tunnel: [TRUE FALSE] -> w861
          frame False {
          }
          frame True {
            n468 = One Button Dialog(message="Insert file name!") -> ()  [unwired: 1 in, 1 out]
          }
        }
        n469 = String To Path(string=w872) -> (path=w871:path)
        n470 = Equal?(x=w867, y=-1) -> (x = y?=w865:bool)
        n471 = case shown="False" w865 {
          selector: w865 -> [_ w921]
          tunnel: [w919 w921] -> w862
          frame False {
            n472 = Two Button Dialog(message="A file with this name already exists!\nDo you want to overwrite?") -> (T button?=w919:bool)  [unwired: 2 in]
          }
          frame True {
          }
        }
        n473 = And(x=w862, y=w861) -> (x .and. y?=w860:bool)
        n474 = case shown="True" w860 {
          tunnel: w871 -> [_ w879]
          frame False {
          }
          frame True {
            n475 = local read "Cycle Pattern"() -> (w878:string[][])
            n476 = call "Table check.vi"("Input table"=w878) -> ("Incomplete?"=w876:bool, "Length"=w877:i32)  [unwired: 9 in]
            n477 = case shown="False" w876 {
              tunnel: w879 -> [w888 _]
              tunnel: w878 -> [w887 _]
              tunnel: w877 -> [w880 _]
              frame False {
                n478 = Number To Decimal String(number=w880) -> (decimal integer string=w883:string)  [unwired: 1 in]
                n479 = for {
                  N: w880 -> [_]
                  tunnel: w887 -> [w917]
                  shift-right: [w905] -> w884
                  shift-left: string[] [] -> [w915]
                  i -> [w916]
                  w896 = 12 ("length")
                  n480 = Index Array(array=w917, index (row)=w916) -> (element=w911:string[])  [unwired: 1 in]
                  n481 = Index Array(array=w911, index=3) -> (element=w901:string)
                  n482 = Index Array(array=w911, index=1) -> (element=w900:string)
                  n483 = Concatenate Strings("C:\\Setup Files\\Subcycles Folder\\", w900) -> (w912:string)
                  n484 = String To Path(string=w912) -> (path=w913:path)
                  n485 = call-poly <vilib>:"Read From Spreadsheet File.vi"("file path (dialog if empty)"=w913) -> ("first row"=w904:string[])  [unwired: 6 in, 4 out]
                  n486 = Delete From Array(array=w904, length=1, index=0) -> (array with subset deleted=w898:string[])  [unwired: 1 out]
                  n487 = String Length(string=w898) -> (length=w907:i32[])
                  n488 = Array Size(array=w907) -> (size(s)=w899:i32)
                  n489 = Divide(x=w899, y=w896) -> (x/y=w897:dbl)
                  n490 = Decrement(x=w897) -> (x-1=w889:dbl)
                  n491 = Multiply(x=w896, y=w889) -> (x*y=w895:dbl)
                  n492 = Number To Decimal String(number=w889) -> (decimal integer string=w906:string)  [unwired: 1 in]
                  n493 = Delete From Array(array=w898, length=12, index=w895) -> (deleted portion=w892:string[], array with subset deleted=w893:string[])
                  n494 = Index Array(array=w892, index=0) -> (element=w890:string)
                  n495 = Build Array (concatenate)(w900, w901, w906, w890, w893) -> (w910:string[])
                  n496 = Build Array (concatenate)(w915, w910) -> (w905:string[])
                }
                n497 = local write "Flag 2"(FALSE) -> ()
                n498 = Build Array (concatenate)("Cycle Data File for EYECAT - do not modify", w883, w884) -> (w885:string[])
                n499 = call-poly <vilib>:"Write To Spreadsheet File.vi"("1D data"=w885, "file path (dialog if empty)"=w888) -> ()  [unwired: 6 in, 1 out]
              }
              frame True {
                n500 = One Button Dialog(message="The table is incomplete!\nplease review and save again!") -> ()  [unwired: 1 in, 1 out]
              }
            }
          }
        }
      }
      frame "load cycle" {
        n501 = local read "Flag 2"() -> (w925:bool)
        n502 = case shown="True" w925 {
          tunnel: [w964 w966] -> w922
          tunnel: w924 -> [w964 w966]
          tunnel: [TRUE ("T button?") w965] -> w923
          frame False {
          }
          frame True {
            n503 = Two Button Dialog(message="The table has been modified.\nDo you want to continue?") -> (T button?=w965:bool)  [unwired: 2 in]
          }
        }
        n504 = case shown="True" w923 {
          tunnel: w922 -> [_ w928]
          frame False {
          }
          frame True {
            n505 = property on="Cycle List" class="LstBox (strict)"() -> ("Item Names"=w944:string[])  [unwired: 2 in, 2 out]
            n506 = Index Array(array=w944, index="Cycle List") -> (element=w930:string)
            n507 = Concatenate Strings(w928, w930) -> (w943:string)
            n508 = Search/Split String(string=w930, search string/char (-)=".") -> (substring before match=w929:string)  [unwired: 1 in, 2 out]
            n509 = String To Path(string=w943) -> (path=w942:path)
            n510 = local write "Cycle Name"(w929) -> ()
            n511 = call-poly <vilib>:"Read From Spreadsheet File.vi"("file path (dialog if empty)"=w942) -> ("first row"=w926:string[])  [unwired: 6 in, 4 out]
            n512 = Delete From Array(array=w926, length=2, index=0) -> (array with subset deleted=w927:string[])  [unwired: 1 out]
            n513 = Index Array(array=w926, index=1) -> (element=w941:string)
            n514 = Decimal String To Number(string=w941) -> (number=w940:i32)  [unwired: 2 in, 1 out]
            n515 = for {
              N: w940 -> [_]
              tunnel: w927 -> [w962]
              tunnel: [w957] -> w935 mode=indexing
              shift-right: [w947] -> _
              shift-left: 0 ("x") -> [w948]
              i -> [w961]
              w958 = ""
              n516 = Increment(x=w948) -> (x+1=w946:i32)
              n517 = Increment(x=w946) -> (x+1=w954:i32)
              n518 = Increment(x=w961) -> (x+1=w956:i32)
              n519 = Number To Decimal String(number=w956) -> (decimal integer string=w955:string)  [unwired: 1 in]
              n520 = Index Array(array=w962, index #1=w948, index #2=w946, index #3=w954) -> (element #1=w960:string, element #2=w959:string, element #3=w953:string)
              n521 = Build Array(w955, w960, w958, w959, w958) -> (w957:string[])
              n522 = Decimal String To Number(string=w953) -> (number=w952:i32)  [unwired: 2 in, 1 out]
              n523 = Multiply(x=w952, y=12 ("x")) -> (x*y=w950:i32)
              n524 = Compound Arithmetic op=ADD(w950, 4, w948) -> (w947:i32)
            }
            n525 = Insert Into Array(array=string[][] [["", "", "", "", ""], ["", "", "", "", ""], ["", "", "", "", ""], ["", "", "", "", ""], ["", "", "", "", ""], ["", "", "", "", ""], ["", "", "", "", ""], ["", "", "", "", ""], ["", "", "", "", ""], ["", "", "", "", ""], ["", "", "", "", ""], ["", "", "", "", ""], ["", "", "", "", ""], ["", "", "", "", ""], ["", "", "", "", ""], ["", "", "", "", ""], ["", "", "", "", ""], ["", "", "", "", ""], ["", "", "", "", ""], ["", "", "", "", ""], ["", "", "", "", ""], ["", "", "", "", ""], ["", "", "", "", ""], ["", "", "", "", ""], ["", "", "", "", ""], ["", "", "", "", ""], ["", "", "", "", ""], ["", "", "", "", ""], ["", "", "", "", ""], ["", "", "", "", ""], ["", "", "", "", ""]], index (row)=0, new element=w935) -> (w934:string[][])  [unwired: 1 in]
            n526 = local write "Cycle Pattern"(w934) -> ()
          }
        }
      }
      frame "delete cycle" {
        n527 = Two Button Dialog(message="This operation will permanently delete this file!\nDo you want to continue?") -> (T button?=w970:bool)  [unwired: 2 in]
        n528 = case shown="True" w970 {
          tunnel: w969 -> [_ w975]
          frame False {
          }
          frame True {
            n529 = local read "Cycle List"() -> (w976:i32)
            n530 = property on="Cycle List" class="LstBox (strict)"() -> ("Item Names"=w977:string[])  [unwired: 2 in, 2 out]
            n531 = Index Array(array=w977, index=w976) -> (element=w974:string)
            n532 = Concatenate Strings(w975, w974) -> (w973:string)
            n533 = String To Path(string=w973) -> (path=w972:path)
            n534 = Delete(path (use dialog)=w972) -> ()  [unwired: 4 in, 3 out]
            n535 = local write "Flag 2"(FALSE) -> ()
          }
        }
      }
      frame "calc HC CO" {
        n536 = local read "Sub-Cycle Pattern"() -> (w994:string[][])
        n537 = Index Array(array=w994, index (col) #1=3 ("disabled index (col)"), index (col) #2=4 ("index (col)"), index (col) #3=11 ("index (col)")) -> (element #1=w984:string[], element #2=w991:string[], element #3=w978:string[])  [unwired: 3 in]
        n538 = Array Size(array=w984) -> (size(s)=w982:i32)
        n539 = Search 1D Array(1D array=w984, element="") -> (index of element=w981:i32)  [unwired: 1 in]
        n540 = Equal?(x=w981, y=-1) -> (x = y?=w983:bool)
        n541 = Select(t=w982, s=w983, f=w981) -> (s? t:f=w980:i32)
        n542 = for {
          N: w980 -> [_]
          tunnel: [w1005] -> w988 mode=indexing
          tunnel: [w1004] -> w987 mode=indexing
          tunnel: w984 -> [w1003] mode=indexing
          tunnel: w991 -> [w1002] mode=indexing
          tunnel: w978 -> [w1001] mode=indexing
          w1000 = ""
          n543 = Not Equal?(x=w1003, y=w1000) -> (x != y?=w999:bool)
          n544 = Not Equal?(x=w1002, y=w1000) -> (x != y?=w998:bool)
          n545 = Not Equal?(x=w1001, y=w1000) -> (x != y?=w997:bool)
          n546 = Compound Arithmetic op=AND(w999, w998, w997) -> (w996:bool)
          n547 = case shown="True" w996 {
            tunnel: w1003 -> [_ w1034]
            tunnel: w1002 -> [_ w1033]
            tunnel: [w1006 w1030] -> w1004
            tunnel: [w1006 w1029] -> w1005
            tunnel: w1001 -> [_ w1007]
            frame False {
              w1006 = ""
            }
            frame True {
              # "O2Eq"
              n548 = Fract/Exp String To Number(string=w1007) -> (number=w1008:dbl)  [unwired: 3 in, 1 out]
              n549 = Fract/Exp String To Number(string=w1034) -> (number=w1015:dbl)  [unwired: 3 in, 1 out]
              n550 = Fract/Exp String To Number(string=w1033) -> (number=w1011:dbl)  [unwired: 3 in, 1 out]
              n551 = Decrement(x=w1015) -> (x-1=w1016:dbl)
              n552 = Divide(x=w1008, y=20000.0) -> (x/y=w1009:dbl)
              n553 = Multiply(x=4.76, y=w1015) -> (x*y=w1020:dbl)
              n554 = Multiply(x=w1016, y=100.0) -> (x*y=w1018:dbl)
              n555 = Add(x=w1011, y=w1009) -> (x+y=w1012:dbl)
              n556 = Add(x=0.33, y=w1020) -> (x+y=w1022:dbl)
              n557 = Divide(x=w1018, y=w1022) -> (x/y=w1023:dbl)
              n558 = Subtract(x=w1012, y=w1023) -> (x-y=w1025:dbl)
              n559 = Multiply(x=w1025, y=2.0) -> (x*y=w1013:dbl)
              n560 = Divide(x=w1025, y=5.0) -> (x/y=w1014:dbl)
              n561 = Number To Fractional String(number=w1014, width (-)=i16 6, precision (6)=i16 3) -> (F-format string=w1029:string)  [unwired: 1 in]
              n562 = Number To Fractional String(number=w1013, width (-)=i16 6, precision (6)=i16 2) -> (F-format string=w1030:string)  [unwired: 1 in]
            }
          }
        }
        n563 = Replace Array Subset(array=w994, new element #1=w988, index (col) #1=5 ("disabled index (col)"), new element #2=w987, index (col) #2=6 ("disabled index (col)")) -> (w992:string[][])  [unwired: 2 in]
        n564 = local write "Sub-Cycle Pattern"(w992) -> ()
      }
      frame "Total time calc" {
        w1049 = i16 2 ("width (-)")
        w1056 = ":"
        n565 = local read "Cycle Pattern"() -> (w1063:string[][])
        n566 = Index Array(array=w1063, index (col)=4 ("disabled index (col)")) -> (element=w1036:string[])  [unwired: 1 in]
        n567 = Array Size(array=w1036) -> (size(s)=w1038:i32)
        n568 = Search 1D Array(1D array=w1036, element="") -> (index of element=w1037:i32)  [unwired: 1 in]
        n569 = Equal?(x=w1037, y=-1) -> (x = y?=w1039:bool)
        n570 = Select(t=w1038, s=w1039, f=w1037) -> (s? t:f=w1035:i32)
        n571 = for {
          N: w1035 -> [_]
          tunnel: w1036 -> [w1071] mode=indexing
          shift-right: [w1073] -> w1059
          shift-left: 0 -> [w1074]
          n572 = xnode "Match Regular Expression"("input string"=w1071, "regular expression"=":" ("search string/char (-)")) -> ("before match"=w1070:string, "after match"=w1067:string)  [unwired: 4 in, 3 out]
          n573 = Decimal String To Number(string=w1070) -> (number=w1069:i32)  [unwired: 2 in, 1 out]
          n574 = Decimal String To Number(string=w1067) -> (number=w1066:i32)  [unwired: 2 in, 1 out]
          n575 = Multiply(x=w1069, y=60) -> (x*y=w1065:i32)
          n576 = Add(x=w1065, y=w1066) -> (x+y=w1064:i32)
          n577 = Add(x=w1064, y=w1074) -> (x+y=w1073:i32)
        }
        n578 = local read "Total Number of Cycles"() -> (w1060:T1)
        n579 = Multiply(x=w1059, y=w1060) -> (x*y=w1055:T1)
        n580 = Quotient & Remainder(x=w1055, y=3600.0) -> (x-y*floor(x/y)=w1042:T1, floor(x/y)=w1052:T1)
        n581 = Quotient & Remainder(x=w1042, y=60.0) -> (x-y*floor(x/y)=w1050:T1, floor(x/y)=w1051:T1)
        n582 = Number To Decimal String(number=w1052) -> (decimal integer string=w1057:string)  [unwired: 1 in]
        n583 = Number To Decimal String(number=w1051, width (-)=w1049) -> (decimal integer string=w1053:string)
        n584 = Number To Decimal String(number=w1050, width (-)=w1049) -> (decimal integer string=w1048:string)
        n585 = Concatenate Strings(w1057, w1056, w1053, w1056, w1048) -> (w1047:string)
        n586 = call <vilib>:"Search and Replace Pattern.vi"("string"=w1047, "regular expression (\"\")"=" " ("replace string (\"\")"), "replace string (\"\")"="0" ("replace string (\"\")"), "replace all? (F)"=TRUE) -> ("result string"=→"Total Test Duration (hrs)":string)  [unwired: 1 in, 1 out]
      }
      frame "update Cycle pattern " {
        n587 = local read "Cycle Pattern"() -> (w1202:string[][])
        n588 = Index Array(array=w1202, index (col)=1 ("disabled index (col)")) -> (element=w1187:string[])  [unwired: 1 in]
        n589 = String To Path(string=w1204) -> (path=w1205:path)
        n590 = Array Size(array=w1187) -> (size(s)=w1190:i32)
        n591 = Search 1D Array(1D array=w1187, element="") -> (index of element=w1189:i32)  [unwired: 1 in]
        n592 = List Folder(path=w1205, pattern="*.eyes") -> (filenames=w1203:string[])  [unwired: 2 in, 3 out]
        n593 = Equal?(x=w1189, y=-1) -> (x = y?=w1191:bool)
        n594 = Select(t=w1190, s=w1191, f=w1189) -> (s? t:f=w1188:i32)
        n595 = for {
          N: w1188 -> [_]
          tunnel: w1202 -> [w1221] mode=indexing
          tunnel: w1204 -> [w1214]
          tunnel: [w1216] -> w1197 mode=indexing
          tunnel: [w1218] -> w1201 mode=indexing
          tunnel: [w1215] -> w1198 mode=indexing
          tunnel: w1203 -> [w1213]
          tunnel: [w1208] -> w1194 mode=indexing
          n596 = Index Array(array=w1221, index #1=1 ("index"), index #2=3 ("index")) -> (element #1=w1212:string, element #2=w1217:string)
          n597 = Search 1D Array(1D array=w1213, element=w1212) -> (index of element=w1211:i32)  [unwired: 1 in]
          n598 = Not Equal?(x=w1211, y=-1) -> (x != y?=w1209:bool)
          n599 = case shown="True" w1209 {
            tunnel: [w1225 w1239] -> w1218
            tunnel: w1217 -> [_ w1235]
            tunnel: [w1225 w1233] -> w1216
            tunnel: [w1225 w1232] -> w1215
            tunnel: w1214 -> [_ w1231]
            tunnel: w1212 -> [w1224 w1230]
            tunnel: [w1223 w1230] -> w1208
            frame False {
              w1225 = "N/A" ("String")
              n600 = Concatenate Strings(w1224, " - File NOT AVAILABLE !!!" ("string")) -> (w1223:string)
            }
            frame True {
              w1243 = i16 2 ("width (-)")
              n601 = Concatenate Strings(w1231, w1230) -> (w1261:string)
              n602 = String To Path(string=w1261) -> (path=w1260:path)
              n603 = call <vilib>:"Search and Replace Pattern.vi"("string"=w1235, "regular expression (\"\")"="[a-x ]" ("format string"), "replace string (\"\")"="", "replace all? (F)"=TRUE) -> ("result string"=w1232:string)  [unwired: 1 in, 1 out]
              n604 = call-poly <vilib>:"Read From Spreadsheet File.vi"("file path (dialog if empty)"=w1260) -> ("first row"=w1229:string[])  [unwired: 6 in, 4 out]
              n605 = Delete From Array(array=w1229, length=1, index=0) -> (array with subset deleted=w1228:string[])  [unwired: 1 out]
              n606 = Array Size(array=w1228) -> (size(s)=w1259:i32)
              n607 = Equal?(x=w1232, y="") -> (x = y?=w1247:bool)
              n608 = Subtract(x=w1259, y=12) -> (x-y=w1257:i32)
              n609 = Select(t="0", s=w1247, f=w1232) -> (s? t:f=w1246:string)
              n610 = Index Array(array=w1228, index=w1257) -> (element=w1233:string)
              n611 = Decimal String To Number(string=w1246) -> (number=w1256:i32)  [unwired: 2 in, 1 out]
              n612 = Decimal String To Number(string=w1233) -> (number=w1255:i32)  [unwired: 2 in, 1 out]
              n613 = Multiply(x=w1256, y=w1255) -> (x*y=w1254:i32)
              n614 = Quotient & Remainder(x=w1254, y=60) -> (x-y*floor(x/y)=w1252:i32, floor(x/y)=w1251:i32)
              n615 = Number To Decimal String(number=w1252, width (-)=w1243) -> (decimal integer string=w1249:string)
              n616 = Number To Decimal String(number=w1251, width (-)=w1243) -> (decimal integer string=w1248:string)
              n617 = Concatenate Strings(w1248, ":", w1249) -> (w1242:string)
              n618 = call <vilib>:"Search and Replace Pattern.vi"("string"=w1242, "regular expression (\"\")"=" " ("replace string (\"\")"), "replace string (\"\")"="0" ("replace string (\"\")"), "replace all? (F)"=TRUE) -> ("result string"=w1239:string)  [unwired: 1 in, 1 out]
            }
          }
        }
        n619 = Replace Array Subset(array=w1202, new element #1=w1194, index (col) #1=1 ("disabled index (col)"), new element #2=w1197, index (col) #2=2 ("disabled index (col)"), new element #3=w1198, index (col) #3=3 ("disabled index (col)"), new element #4=w1201, index (col) #4=4 ("disabled index (col)")) -> (w1206:string[][])  [unwired: 4 in]
        n620 = local write "Cycle Pattern"(w1206) -> ()
      }
      frame "load cycle name" {
        n621 = property on="Cycle Pattern" class="Tbl (strict)"() -> ("EditPos"=w1267:T3)  [unwired: 2 in, 2 out]
        n622 = Unbundle By Name(w1267) -> ("Row"=w1265:i32, "Column"=w1264:i32)
        n623 = local read "Cycle Pattern"() -> (w1263:string[][])
        n624 = call "SubCycles list.vi"() -> ("Subcycle name"=w1266:string)  [unwired: 10 in, 1 out]
        n625 = Replace Array Subset(array=w1263, new element=w1266, index (row)=w1265, index (col)=w1264) -> (w1262:string[][])
        n626 = local write "Cycle Pattern"(w1262) -> ()
      }
      frame "load test array" {
        n627 = local read "Total Test Duration (hrs)"() -> (w1275:T8)
        n628 = local read "Cycle Name"() -> (w1271:T5)
        n629 = Equal?(x=w1271, y="") -> (x = y?=w1270:bool)
        n630 = Not Equal?(x=w1275, y="0:00:00") -> (x != y?=w1269:bool)
        n631 = Or(x=w1269, y=w1270) -> (x .or. y?=w1268:bool)
        n632 = case shown="True" w1268 {
          selector: w1268 -> [w1276 _]
          tunnel: [FALSE TRUE] -> w1273
          frame False {
            n633 = case shown="False" w1276 {
              frame False {
                n634 = One Button Dialog(message="Incomplete Data!\nReview the cycle pattern!") -> ()  [unwired: 1 in, 1 out]
              }
              frame True {
              }
            }
          }
          frame True {
            w1282 = 0.0 ("default (0 I32)")
            n635 = local read "Cycle Name"() -> (w1297:T5)
            n636 = Concatenate Strings("C:\\Setup Files\\Cycles Folder\\", w1297, ".eyec" ("string")) -> (w1295:string)
            n637 = String To Path(string=w1295) -> (path=w1296:path)
            n638 = local read "Total Number of Cycles"() -> (w1293:T1)
            n639 = call-poly <vilib>:"Read From Spreadsheet File.vi"("file path (dialog if empty)"=w1296) -> ("first row"=w1279:string[])  [unwired: 6 in, 4 out]
            n640 = call "Remove names.vi"("Array in"=w1279) -> ("Array out"=w1288:string[])  [unwired: 10 in]
            n641 = Index Array(array=w1279, index #1=14 ("index"), index #2=15 ("index")) -> (element #1=w1284:string, element #2=w1280:string)
            n642 = Number To Decimal String(number="Ageing Gas") -> (decimal integer string=w1292:string)  [unwired: 1 in]
            n643 = Number To Decimal String(number=w1293) -> (decimal integer string=w1291:string)  [unwired: 1 in]
            n644 = Decimal String To Number(string=w1280, default (0L)=w1282) -> (number=w1281:dbl)  [unwired: 1 in, 1 out]
            n645 = Decimal String To Number(string=w1284, default (0L)=w1282) -> (number=w1283:dbl)  [unwired: 1 in, 1 out]
            n646 = property on="Inlet temp Age" class="DigNum (strict)"("Value"=w1283) -> ()  [unwired: 2 in, 2 out]
            n647 = property on="Flow rate Age" class="DigNum (strict)"("Value"=w1281) -> ()  [unwired: 2 in, 2 out]
            n648 = Build Array (concatenate)(w1292, w1291, w1288) -> (w1287:string[])
            n649 = shared-variable "cRIO-9082\\Library 1.lvlib\\Ageing Variables"(w1287) -> ()  [unwired: 1 in, 1 out]
          }
        }
        "Test Compiled" <- w1273
      }
      frame "convert to num" {
        n650 = local read "EditPos Subc"() -> (w1302:T3)
        n651 = Unbundle By Name(w1302) -> ("Row"=w1303:i32, "Column"=w1300:i32)
        n652 = Equal?(x=w1300, y=7) -> (x = y?=w1299:bool)
        n653 = case shown="False" w1299 {
          tunnel: w1303 -> [_ w1308]
          tunnel: w1300 -> [_ w1306]
          tunnel: w1302 -> [_ _]
          frame True {
          }
          frame False {
            n654 = local read "Sub-Cycle Pattern"() -> (w1305:string[][])
            n655 = call "Conv to num.vi"("Column"=w1306, "Row"=w1308, "Array"=w1305) -> ("result string"=w1307:string)  [unwired: 8 in]
            n656 = Replace Array Subset(array=w1305, new element=w1307, index (row)=w1308, index (col)=w1306) -> (w1304:string[][])
            n657 = local write "Sub-Cycle Pattern"(w1304) -> ()
          }
        }
      }
      frame "check scycle name" {
        n658 = local read "Sub-Cycle Name"() -> (w1309:T5)
        n659 = call <vilib>:"Search and Replace Pattern.vi"("string"=w1309, "regular expression (\"\")"="[^0-9a-zA-Z ]" ("format string"), "replace string (\"\")"="", "replace all? (F)"=TRUE) -> ("result string"=w1315:string)  [unwired: 1 in, 1 out]
        n660 = Not Equal?(x=w1315, y=w1309) -> (x != y?=w1314:bool)
        n661 = case shown="False" w1314 {
          tunnel: w1315 -> [w1316 w1317]
          tunnel: [w1316 w1317] -> w1310
          frame False {
          }
          frame True {
            n662 = One Button Dialog(message="Unsuitable character for the file name!") -> ()  [unwired: 1 in, 1 out]
          }
        }
        n663 = local write "Sub-Cycle Name"(w1310) -> ()
      }
      frame "check cycle name" {
        n664 = local read "Cycle Name"() -> (w1319:T5)
        n665 = call <vilib>:"Search and Replace Pattern.vi"("string"=w1319, "regular expression (\"\")"="[^0-9a-zA-Z ]" ("format string"), "replace string (\"\")"="", "replace all? (F)"=TRUE) -> ("result string"=w1325:string)  [unwired: 1 in, 1 out]
        n666 = Not Equal?(x=w1325, y=w1319) -> (x != y?=w1324:bool)
        n667 = case shown="False" w1324 {
          tunnel: w1325 -> [w1326 w1327]
          tunnel: [w1326 w1327] -> w1320
          frame False {
          }
          frame True {
            n668 = One Button Dialog(message="Unsuitable character for the file name!") -> ()  [unwired: 1 in, 1 out]
          }
        }
        n669 = local write "Cycle Name"(w1320) -> ()
      }
      frame "Multigas connect" {
        # "add here logic to verify the user requirements and the machine state\n0 - not connected\n1 - MKS1 & Ext An Up\n2 - MKS2 & Ext An Dn\n3 - MKS 1 & 2  & Ext An Up & Dn"
        n670 = flat-sequence {
          frame #0 {
            "Connected?" <- TRUE
          }
        }
      }
      frame "Multigas disconnect" {
      }
    }
    n671 = local read "stop 2"() -> (w709:bool)
  }
  n672 = node-c288(w1) -> ()  [unwired: 1 out]
  n673 = local write "stop 2"(w11) -> ()
  n674 = disable-structure shown="Disabled" {
    frame Disabled {
      n675 = while {
        tunnel: [w1368] -> w1353
        tunnel: [w1367] -> w1352
        stop <- w1364 stop-if-true
        n676 = TCP Open Connection(address="192.168.1.3", remote port or service name=u16 7700) -> (connection ID=w1368:refnum<k5>, error out=w1367:errorcluster)  [unwired: 3 in]
        n677 = Unbundle By Name(w1367) -> ("status"=w1369:bool)
        n678 = Not(x=w1369) -> (.not. x?=w1365:bool)
        n679 = Or(x=w1365, y="stop TCP") -> (x .or. y?=w1364:bool)
      }
      n680 = Concatenate Strings("\r", "\n") -> (w1341:string)
      n681 = Concatenate Strings("MSSM,0,1,1" ("data in"), w1341) -> (w1348:string)
      n682 = TCP Write(connection ID=w1353, data in=w1348, error in (no error)=w1352) -> (connection ID out=w1356:refnum<k5>, error out=w1357:errorcluster)  [unwired: 1 in, 1 out]
      n683 = Concatenate Strings("MSMD,1,7,1,1,1,1,2,1,1,3,1,1,4,1,1,5,1,1,6,1,1,7,1" ("data in"), w1341) -> (w1343:string)
      n684 = TCP Write(connection ID=w1356, data in=w1343, error in (no error)=w1357) -> (connection ID out=w1354:refnum<k5>, error out=w1355:errorcluster)  [unwired: 1 in, 1 out]
      n685 = Concatenate Strings("MSTT,1,0" ("string"), w1341) -> (w1342:string)
      n686 = TCP Write(connection ID=w1354, data in=w1342, error in (no error)=w1355) -> (connection ID out=w1340:refnum<k5>, error out=w1339:errorcluster)  [unwired: 1 in, 1 out]
      n687 = UDP Open(9:500 ("timeout ms (25000)"), 11:u16 7701 ("port")) -> ()  [unwired: 3 in, 3 out]
      n688 = UDP Read(timeout ms (25000)=500) -> (data out=w1331:string)  [unwired: 3 in, 4 out]
      n689 = while {
        shift-right: [w1360] -> _
        shift-left: w1331 -> [w1363]
        tunnel: [w1361] -> w1332 mode=indexing
        stop <- w1358 stop-if-true
        n690 = Search/Split String(string=w1363, search string/char (-)=",") -> (substring before match=w1361:string, match + rest of string=w1360:string)  [unwired: 1 in, 1 out]
        n691 = String Length(string=w1360) -> (length=w1359:i32)
        n692 = Equal To 0?(x=w1359) -> (x = 0?=w1358:bool)
      }
      n693 = call "7170string to array.vi"("Array in"=w1332) -> ()  [unwired: 4 in, 1 out]
      n694 = UDP Close() -> ()  [unwired: 2 in, 2 out]
      n695 = Concatenate Strings("MSTP,0,0" ("string"), "\r", "\n") -> (w1335:string)
      n696 = TCP Write(data in=w1335) -> (connection ID out=w1337:refnum<k5>, error out=w1338:errorcluster)  [unwired: 3 in, 1 out]
      n697 = TCP Close Connection(connection ID=w1337, error in (no error)=w1338) -> ()  [unwired: 1 in, 2 out]
    }
    frame Enabled {
    }
  }
  n698 = node-c288(w8) -> ()  [unwired: 1 out]
  "Table" <- string[][] [] ("Table")
